vi "Argos 2.0.vi"(0 "PID 1 COM":refnum<visa-resource-name>="COM1", 1 "Setpoint\n START":bool, 2 "Write to File":bool, 3 "SP 1 input (°C)":dbl=10.0 min=0.0 max=1300.0, 4 "Intervall (s)":u32=1 max=600, 5 "Write/\nRead":bool=TRUE, 6 "Delay (ms)":u32=500 min=100 max=600000, 7 "Auto Tune":bool, 9 "Standby":bool, 11 "Reset\nSTOP":bool, 12 "ON":bool=TRUE caption="OFF", 13 "Get Values":bool, 15 "File Path":path) -> (8 "(°C)":dbl format="%#.3f", 14 "SP 1 is (°C)":dbl)   [LabVIEW 2013]
doc: "1. Verwendung\n\nDas Programm dient der Steuerung und Abfrage des Thermocontrollers I3252 und dem Auslesen von zwei VC 840 Messgeräten und einem Druckmessgerät Pfeiffer Single Gauge. \nDie Messgeräte werden Standardmäßig ausgelesen und erst nach Betätigung des Schalters \"Write to File\" in einer Textdatei abgespeichert. Das Eingabefeld \"Intervall\" legt den Abstand der Messpunkte fest.\nDer Setpoint für den Thermocontroller wird erst nach Betätigung des Tasters \"Setpoint START\" übernommen und angesteuert. Er wird ind den EEPROM des Gerätes geschrieben. Die Regelung kann mit Hilfe des Schalters \"Standby\" unterbrochen werden. Durch den Taster \"Reset STOPP\" kann der Setpoint aus dem EEPROM gelöscht werden.\nDie Eingabeflächen \"Constant\" und \"Thickness\" dienen der Berechnung des spezifischen Widerstands.\nDie Eingabeflächen \"User\" und \"Sample\" werden in den Header der Textdatei übernommen.\nDer Indikator \"File Path\" zeigt den aktuellen Speicherort der Textdatei an. Dieser wird nach ausschalten des Schalters \"Write to File\" gelöscht. Bei erneuten Schreiben muss ein neuer Speicherort gewählt werden. Bei Wahl desselben Speicherorts werden sämtliche bereits gespeicherte Daten gelöscht.\n\n\n2. Erläuterungen zum Blockdiagramm\n2.1 äußere Sequenz\nDie äußerte Sequenz besteht aus fünf Frames. Der erste dient der Initialisierung der Ports. Der zweite dient als Verzögerung um dem Programm genug Zeit zu geben die Ports zu öffnen. Jedoch senden die beiden VC 840 bereits Informationen an den Computer die in einem Puffer zwischengespeichert werden. Im dritten Frame wird dieser Puffer geleert. Somit kommt es zu keinem Framing Error. Desweiteren wird in diesem Frame die Startzeit der Messungen genommen. Im vierten Frame wird die eigentliche Messung und Verarbeitung der Daten durchgeführt. Die while-Schleife wird nur durch Auftreten eines Fehlers oder durch Betätigung des Stopbuttons auf dem Front Panel in der oberen linken Ecke unterbrochen. Im fünften und letzten Frame werden die Ports wieder geschlossen und beim Auftreten eines Fehlers wird das Programm automatisch gestoppt. Falls kein Fehler auftritt wird die Sequenz von vorne abgearbeitet.\n\n2.2 while-Schleife und innere Sequenz\n2.2.1 \"Event Structure\"\n2.2.1.1 Allgemein\nDer erste Frame beinhaltet ein \"Event Structure\". Dieser reagiert auf insgesamt elf verschiedene Ereignisse. Falls keines dieser Ereignisse auftreten sollte, warte die Struktur eine Millisekunde bevor die \"Event Structure\" verlassen wird. Die übrigen Ereignisse treten ein, wenn der entsprechende Kontroller eine Werteänderung erfährt.\n\n2.2.1.2 Event: Setpoint\nDieser Case besteht von außen nach innen aus einer Stacked Sequence, einer for-Loop und einer Flat Sequence die wiederum zwei \"Case Structures\" enthält. Als erstes wird bei dem Schalter \"Setpoint START\" der Blinkmodus aktiviert und bei dem Schalter \"Read Temperature\" deaktiviert. Danach folgt das eigentliche setzen des Temperatursollwerts. In der ersten Iteration wird dem Controller I3252 ein Schreibbefehl gesendet. Theoretisch kann der Setpoint in den RAM oder in den EEPROM geschrieben werden. Diese Auswahl erfolgt mit Hilfe des Schalters \"RAM\". Da das Schreiben in den RAM -Speicher aber aus diversen Gründen nicht erwünscht ist, wurde es nicht implementiert. Eine nachträgliche Implementierung ist aber leicht möglich, in dem die untere String-Konstante \"*P012\" durch \"*W012\" ersetzt wird. An diesem Befehl wird eine fünfstellige Hexadezimalzahl angehängt, die den Sollwert wiedergibt. Der Sollwert wird vorher mit zehn multipliziert, da das Komma standardmäßig nach der ersten Ziffer festgesetzt wurde (Bsp.: 800 wird gesendet um 80 einzustellen). Dieser Befehlsstrang wird an das Gerät mittels des SubVIs \"Comm_Interface\", auf welches später noch näher eingegangen wird, weitergegeben. Der durch das Gerät zurückgegebene String wird nicht verarbeitet.\nDie zweite Iteration dient dem Auslesen des eingestellten Sollwertes. Wahlweise kann der RAM- oder der EEPROM-Speicher ausgelesen werden. Die eigentliche Verarbeitung des Ausgabestrings erfolgt durch das SubVI \"Edit Setpoint\".\nDie Implementierung zur Einstellung des zweiten Setpoints erfolgt durch kopieren der ersten beiden Fälle und ersetzen der \"1\" im Befehf durch eine \"2\" (Bsp.: \"*P012\" zu \"*P022\"). Es darf aber nicht vergessen werden, dass dann ebenfalls die Anzahl der Iterationen angepasst werden muss.\nAls letztes wird der Blinkmodus des Schalters \"Setpoint START\" wieder deaktiviert.\n\n2.2.1.3 Event: Standby\nDieses Ereignis aktiviert bzw. deaktiviert als erstes den Blinckmodus des entsprechenden Schalters und sendet danach den Befehl zum aktivieren (\"*D03\") oder zum deaktivieren (\"*E03\") des Standbymodus an den Thermocontroller.\n\n2.2.1.4 Event: Set Command \nDer in das Feld \"Command shall be\" eingegebene Befehl wird an den Thermocontroller übermittlet. Die korrekte Form des Befehls ist im \"Communication Manuel\" nachzuschlagen. Das \"*\"-Zeichen wurde allerdings schon implementiert und muss somit nicht mit eingegeben werden.\n\n2.2.1.5 Event: Reset\nIn der ersten Iteration wird der Reset-Befehl an den Thermocontroller gesendet. In Folge wird der gesamte EEPROM-Speicher gelöscht. Deshalb wird in der zweiten Iteration der Setpoint aktualisiert. Dieser Befehl hat keinen Einfluss auf den RAM-Speicher. Die anschließende Wartezeit ist auf vier Sekunden festgesetzt und wurde empirisch ermittelt. Diese Zeit benötigt das Gerät um den Reset durchzuführen und für die Kommunikation wieder zur Verfügung zu stehen.\n\n2.2.1.6 Event: Auto Tune\nEs ist festgeschrieben, dass der Setpoint für die \"Auto Tune\"-Funktion wenigstens 20°C über der aktuellen Temperatur liegt. Deshalb wird zunächst der aktuelle Temperaturwert ausgelesen. Im zweiten Schritt werden zu diesem Wert zwanzig addiert und der Setpoint wird in den RAM-Speicher geschrieben. Das Schreiben in diesen Speicher ist nötig, da die \"Auto Tune\"-Funktion\" erst nach einem Reset startet. Im dritten Schritt wird der eigentliche Befehl für den \"Auto Tune\" gesendet (siehe dazu \"Communication Manuel\" S.27). Als vierte und letzte Iteration der for-Schleife folgt der bereits erwähnte Reset-Befehl. Der Temperatursollwert, der im RAM-Speicher eingetragen ist, muss zum Schluss wieder auf 0°C gesetzt werden. Die Zeit für die Ausführung des \"Auto Tune\"-Befehls wurde empirisch ermittelt und 45 s festgesetzt.\n\n2.2.1.7 Event: Write LOW/HI\nDieses Ereignis setzt die am Analogausgang anliegende Spannung fest. Normalerweise beträgt dieser Spannungswert 0-10 V. Das angeschlossene Netzteil verträgt aber maximal nur 2,3 V. Aus diesem Grund wird der \"%HIGH\" auf 23 gesetzt. Somit beträgt die maximal anliegende Spannung nur noch 23% von der maximal möglichen, d.h 2,3V. Ein niedrigerer Wert ist jederzeit möglich, genauso wie ein höherer für den Parameter \"%LOW\". Diese werden zunächst nacheinander in den RAM-Speicher geschrieben und anschließend wieder ausgelesen.\n\n2.2.1.8 Event: Set PID\nDie Werte für den PID-Regler können sowohl mit Hilfe der \"Auto Tune\"-Funktion, als auch manuell eingestellt werden. Es wird wiederum zwischen dem Schreiben in den RAM- und dem EEPROM-Speicher unterschieden. Zunächst werden die Werte für \"P\", \"I\" und \"D\", in dieser Reihenfolge, gesetzt und danach die aktuellen Werte ausgelesen.\n\n2.2.1.9 Event: Get Values\nDieses Ereignis hat zur Folge, dass die Werte für \"P\", \"I\", \"D\", \"%LOW\", \"%HIGH\" und des Setpoints wahlweise aus dem RAM- oder EEPROM-Speicher gelesen werden. Die aktuellen Werte werden nicht nur in die entsprechenden Anzeigefelder übernommen, sondern auch in die entsprechenden Eingabefelder, mit Ausnahme des Temperatursollwerts. \n\n2.2.1.10 Event: RAM\nPrinzipiell kann zwischen dem Schreiben in den RAM- oder EEPROM-Speicher des Thermocontrollers gewählt werden. Die entsprechende Schalterposition auf dem Frontpanel zeigt den aktuell verwendeten Speicher an. Die Anzeigewerte werden bei jedem Umschalten aktualisiert und sind im entsprechenden Speicher eingetragen. Die Implementierung ist identisch mit der des Ereignisses \"Get Values\". Es gilt zu beachten, dass die Werte für \"%LOW\" und \"%HIGH\" nur in den RAM-Speicher geschrieben werden können und somit auch nur aus diesem ausgelesen werden können.\n\n2.2.1.11 Event: Set Gauge to Zero\nMit Hilfe der SubVIs \"Get Pressure\" und \"Offset Display\" werden die Werte für den alten und den neuen Offset und der durch den zweiten Drucksensor ermittelt Druck ermittelt. \n\n2.2.1.12 Event: Write to File\nSollte der Schalter \"Write to File\" aktiviert werden, d.h. Schalterposition oben, so wird zunächst durch das SubVI \"Header\" ein Header für die unter \"File Path\" definierte Datei angelegt. Alle Werte, die bereits in der entsprechenden Datei stehen, werden dabei gelöscht.\n\n2.2.2 \"Timed Structures\"\nIm dritten Frame der inneren Sequenz werden die Werte für Zeitpunkt, Temperatur, Spannung, Strom und Druck ermittelt. Damit die Werte zum gleichen Zeitpunkt aufgenommen werden, werden \"Timed Sequences\" eingesetzt. Mit dem entsprechenden Schalter auf dem Front Panel unter dem Tab \"Settings\" kann gewählt werden, ob das entsprechende Gerät ausgelesen werden soll oder nicht. Die einzelnen Sequenzen werden parallel abgearbeitet, womit die Prozesszeit von diesem Frame durch der zeitintensivsten Sequenz abhängt. Dies ist in aller Regel das Auslesen der Temperatur, da ein \"Delay\" von 500 ms oder größer benötigt wird, um den Controller ordentlich ansprechen zu können.\nDie Systemzeit wird durch das SubVI \"System Time in Seconds\" in Sekunden umgerechnet und der in dem Parameter \"Starttime\" gespeicherte Wert wird abgezogen. Somit werden die Sekunden seit dem Start des Programms gezählt.\n\n2.2.3 restlichen Frames\nIm zweiten Frame wird das Intervall zwischen den einzelnen Messwerten festgelegt. Dabei wird der Wert des Parameters \"Delay\" abgezogen. Dieser Wert beträgt im Normalfall 500 ms und ist somit nicht vernachlääsigbar.\nDer Vierte Frame beinhaltet die Umrechnung des Temperatur-Strings in einen Temperaturwert durch das SubVI \"Edit Tmperature\", die Berechnung des spezifischen Widerstands durch das SubVI \"Resistivity Calculation\" und die Überprüfung des Druckwerts. Auch werden die neu gewonnen Werte in das entsprechende Shift-Register übernommen. Falls der Druckwert einen in dem Parameter \"Pressure Limit (mbar)\" festgelegten Grenzwert überschreiten sollte, wird der Thermocontroller automatisch in den Standby-Modus versetzt. Des Weiteren wird der Schalter \"Standby\" solange gesperrt, wie der Druck oberhalb des Grenzwertes liegt. Wenn der Druck wieder unter den Grenzwert gesunken ist, wird der Standby-Befehl nicht automatisch aufgehoben, sondern muss vom Benutzer durch Betätigung des entsprechenden Schalters gegeben werden.\nIm fünften Frame werden die Diagramme erstellt. Dabei wird jedes Mal von neuem das gesamte Shift-Register als Graph dargestellt. Weiterhin werden die Messwerte in ein 1D-Array geschrieben.\nDer sechste und letzte Frame beinhaltet den eigentlich Schreibvorgang der Messwerte in eine Textdatei und die Überprüfung ob ein Fehler vorliegt.\n\n2.3 SubVIs\n2.3.1 Allgemein\nDie SubVIs für die Messgeräte VC840 und das Druckmessgerät wurden aus anderen Quellen übernommen. \n\n2.3.2 \"Header\"\nIn den Header wird zunächst das aktuelle Datum und die aktuelle Zeit übernommen. Die ausgewählte Datei wird dabei überschrieben. Danach wird der Name des Benutzers und der Probe übernommen. Zum Schluss werden die Einheiten in einer Reihe, durch einen Tabulator getrennt, in den Header geschrieben.\n\n2.3.3 \"I3252 Comm Interface\"\nDieses VI stellt die Kommunikation mit dem Thermocontroller her und gibt den Ausgabe-String zurück.\n\n2.3.4 \"I3252 Edit Setpoint\"\nIm Ausgabe-String vom Thermocontroller ist an der vierten Stelle die Stelle des Dezimalpunktes verschlüsselt. Dieses Hexadezimalzahl wird herausgefiltert und an ein \"ENUM Controller\" übergeben. Dieser weist der Hexadezimalzahl eine Nummer zu, mit welcher ein Wert aus einem Array entnommen wird. Dieser Wert dient als Quotient. Der tatsächliche Wert kann somit errechnet werden.\n\n2.3.5 \"I3252 Edit Temperature\"\nDer Temperatur-String, der vom Thermocontroller zurückgegeben wird, wird in eine Dezimalzahl umgewandelt. Manchmal kommt es aus zu Dropouts, die durch dieses Programm herausgefiltert werden. Der letzte Wert wird dabei in einer \"Feedback Node\" gehalten unter der Annahme, dass sich der Temperaturwert nicht sprunghaft ändert.\n\n2.3.6 \"Resistivity Calculation\"\nDer spezifische Widerstand wird nach folgender Formel ausgerechnet. Dabei entspricht t der Dicke der Probe und C ist eine Konstante.\nrho=C*pi*t*U/(ln( 2)*I)\n\n2.3.7 \"System Time in Seconds\"\nZunächst wird die aktuelle Systemzeit ausgelesen. Danach wird diese in Stunden, Minuten und Sekunden aufgeteilt, alles in Sekunden umgerechnet und letztendlich addiert."
uses:
  <vilib>/Platform/TimedLoop/XDataNode/timing_clust.ctl
  <vilib>/Platform/TimedLoop/XDataNode/nitl_modes.ctl
  <vilib>/Platform/TimedLoop/XDataNode/wakeup.ctl
  <vilib>/Instr/_visa.llb/VISA Configure Serial Port (Instr).vi
  <vilib>/Platform/TimedLoop/scheduler/LVUserAPI/_suppVIs/Create_1kHz_TSource.vi
  <vilib>/Utility/file.llb/Write To Spreadsheet File (DBL).vi
  <vilib>/Platform/TimedLoop/XDataNode/XDataNode.xnode
  <vilib>/Platform/TimedLoop/XDataNode/XDNodeRunTimeDep.lvlib
  Dependencies/Pfeiffer TPG261+262 Single+Dual Gauge/Dual Gauge.lvlib
panel:
  out "Thermocouple (Sample holder 1) 2":cluster{dbl[], dbl[]}(graph)
  out "(°C) 2":dbl format="%#.3f"
  out "appended array":dbl[](array[numeric])
  in  "Tab Control":T1(tab)
  out "SP 2 is (°C)":dbl
  in  "SP 2 input (°C)":dbl=10.0 min=0.0 max=1300.0
  in  "Standby\n2":bool
  in  "Setpoint\n START\n2":bool
  out "Pirani (VVP1 Scroll)":cluster{dbl[], dbl[]}(graph)
  in  "Thickness (nm)":dbl min=0.0
  in  "4PP constant":dbl min=0.0 max=5.0
  in  "Sample":string
  in  "User":string
  out "Thermocouple (Sample holder 1)":cluster{dbl[], dbl[]}(graph)
  out "current time (s)":dbl
  out "data logger intervall (s)":dbl
  out "loop time (s)":dbl
  in  "stop":bool
  out "CMR275 Baratron":cluster{dbl[], dbl[]}(graph)
  out "Pressure Baratron 2":dbl format="%#_4e"
  out "PKR251 FullRange":cluster{dbl[], dbl[]}(graph)
  out "Pressure FullRange 2":dbl format="%#_3e"
  out "Pressure Pirani 2":dbl format="%#_3e"
  in  "Reset\nSTOP 2":bool
  out "Pressure OpenPort":cluster{dbl[], dbl[]}(graph)
  out "Pressure OpenPort2":dbl caption="current"
  out "% HIGH Istwert 2":u32
  out "% LOW Istwert 2":u32
  in  "% High Sollwert 2":u32=23 max=24
  in  "% LOW Sollwert 2":u32 max=25
  in  "RAM 2":bool=TRUE caption="EEPROM"
  out "D (Rate) IstWert 2":u32
  out "I ( Reset1) Istwert 2":u32
  out "P (PB1) Istwert 2":u32 caption="actual value"
  in  "D (Rate) Sollwert 2":u32 max=3999
  in  "I ( Reset1) Sollwert 2":u32 max=3999
  in  "P (PB1) Sollwert 2":u32 caption="set value" max=9999
  in  "ON 2":bool=TRUE caption="OFF"
  in  "PID 2 COM":refnum<visa-resource-name>="COM1"
  in  "Delay (ms) 2":u32=500 min=100 max=600000
  in  "Write/\nRead \n\n2":bool=TRUE
  out "status 2":bool caption="Status"
  out "code 2":i32 caption="Code"
  out "code":i32 caption="Code"
  out "status":bool caption="Status"
  in  "Set Gauge to Zero":bool
  out "Status Gauge 1#2":i32(ring) items=["data OK", "underrange", "overrange", "sensor error", "sensor off", "no sensor", "ID error"]
  out "Pressure Gauge 1#2":dbl format="%.3e"
  out "Pressure Gauge 1#1":dbl format="%.3e"
  out "Status Gauge 1#1":i32(ring) items=["data OK", "underrange", "overrange", "sensor error", "sensor off", "no sensor", "ID error"]
  in  "TPG 1 COM":refnum<visa-resource-name>="COM5"
  in  "Pressure Limit (mbar)":dbl=1.0 min=0.0 max=1100.0
  out "Current Offset (mbar)":dbl
  in  "ON (TPG 2)":bool=TRUE caption="OFF"
  in  "ON (TPG 1)":bool=TRUE caption="OFF"
  in  "ON":bool caption="OFF"
  in  "VC 840 2":refnum<visa-resource-name>="COM7"
  out "Reading 2":dbl format="%_4f"
  out "Mode 2":enum16{"?", "Diode", "Beep", "DC", "AC"}(ring)
  out "Unit 2":string
  in  "VC 840 1":refnum<visa-resource-name>="COM7"
  out "Reading 1":dbl format="%_4f"
  out "Mode 1":enum16{"?", "Diode", "Beep", "DC", "AC"}(ring)
  out "Unit 1":string
  out "Status 1":T2
  out "Status 2":T2
  in  "ON":bool caption="OFF"
  out "% HIGH Istwert":u32
  out "% LOW Istwert":u32
  in  "% High Sollwert":u32=23 max=24
  in  "% LOW Sollwert":u32 max=25
  in  "RAM":bool=TRUE caption="EEPROM"
  out "D (Rate) IstWert":u32
  out "I ( Reset1) Istwert":u32
  out "P (PB1) Istwert":u32 caption="actual value"
  in  "D (Rate) Sollwert":u32 max=3999
  in  "I ( Reset1) Sollwert":u32 max=3999
  in  "P (PB1) Sollwert":u32 caption="set value" max=9999
  in  "Set Command":bool
  in  "Set PID":bool
  in  "Write LOW/HI":bool
  out "Command output":string
  in  "Command input":string
  in  "TPG 2 COM":refnum<visa-resource-name>="COM6"
  out "Pressure Gauge 2#2":dbl format="%.3e"
  out "Pressure Gauge 2#1":dbl format="%.3e"
  out "Status Gauge 2#2":i32(ring) items=["data OK", "underrange", "overrange", "sensor error", "sensor off", "no sensor", "ID error"]
  out "Status Gauge 2#1":i32(ring) items=["data OK", "underrange", "overrange", "sensor error", "sensor off", "no sensor", "ID error"]
  out "Command output 2":string
  in  "Command input 2":string
  in  "Set Command\n\n 2":bool
  in  "Auto Tune 2":bool
  in  "Set PID 2":bool
  in  "Write LOW/HI 2":bool
  in  "Get Values 2":bool
  out "Current":cluster{dbl[], dbl[]}(graph)
  out "Voltage":cluster{dbl[], dbl[]}(graph)
  out "Voltage (V)":dbl format="%.4e"
  out "Current (A)":dbl format="%.4e"
  out "Resistivity":cluster{dbl[], dbl[]}(graph)
  out "Resistivity (Ohm*cm)":dbl format="%.3e"
  # "PID 1"
  # "set \nvalue"
  # "actual \nvalue"
  # "T (°C)"
  # "PID 2"
  # "mbar"
  # "Set \nValue\n2"
  # "Actual \nvalue 2"
  # "T (°C)"
  # "mbar"
  # "mbar"
  # "mbar"
  # "Pressure Measurement \n(Pfeiffer TPG261)"
  # "PID Controller (Omega Newport i3252)"
  # "PID Controller 2 (Omega Newport i3252)"
  # "P"
  # "I"
  # "D"
  # "% Low"
  # "% High"
  # "Multimeter\n#1 (VC 840)"
  # "Multimeter\n#2 (VC 840)"
  # "P"
  # "I"
  # "D"
  # "% Low"
  # "% High"
  # "Authors:  Daniel Schuster (sir-dan@web.de)\n                 Steffen Cornelius (s.cornelius@hzdr.de)\n                 Nico Spahn (x)\n\n                 premade SubVIs for readout of Pfeiffer gauge and VC840 Multimeters were used\n                 SubVI \"I3252_Comm_Interface\" is based on a modified Labview example\n\nRelease:  v1.0    \n\nVersion History:\n\nv1.1  -    28.06.2011\n             - Format des Files geändert von %.3f auf %g\n             - maximale Eingabewerte für PID begrenzt\nv1.2  -    12.07.2011\n             - Anzeige p,rho, U, V auf Scientific geändert\n             - y-Achse p,rho auf Log geändert\n             - numerische Zeitanzeige hinzugefügt\n             - 4PP Constant: pi/ln(2)=4,532 set as the default value\nv1.3  -    25.07.2011\n             - Zeitvariable auf EXT geändert, um Sprünge in Diagrammen loszuwerden\nv1.4  -   27.07.2011\n             - ALLE Variablen auf DBL zurückgesetzt wegen Formatierungsproblem im File\n             - Zeitberechnung neu gemacht (Tick count differenzen) -> Zeitsprünge korrigiert ?\n             - Delay/Intervall überarbeitet\nv1.5  -   05.12.2012\n                - Austausch der alten Pfeifer SubvIs durch neue -> nun alle 4 Kanäle des DualGauge\n                                                                                                         Controllers gleichzeitig auslesbar\n                - neue Pfeiffer SubVIs verwendet in Druckwertauslesung und Offset Berechnung des Baratron\n                  Druckes (COM5 Sensor1)\n                - Neuarragement des GUI -> FullRange und Baratron neben Temperatur auf Haupseite zu sehen\n                                                                   Pirani und OpenPort auf Meas.2 zu sehen\n                                                                   Diagnose Seite umfasst nun auch Widerstandsdiagramm\n                - Änderungen der Settingseite -> nun alle 4 Drucksensoren mit aktuellem Messwert und Gerätestatus\n                                                                           zu sehen\n                - The readout of the PID-Temperature Controller and the VC840 Multimeters was not modified\nv1.73  -  18.10.2013\n                - Layout Änderungen\nv.1.8   -  19.01.2014\n                - Änderung Layout Settings Tab\n                - Trennung der beiden TPG Dual Gauge Controls\n                -"
  # "Version 1.73    - last change 18.10.2013"
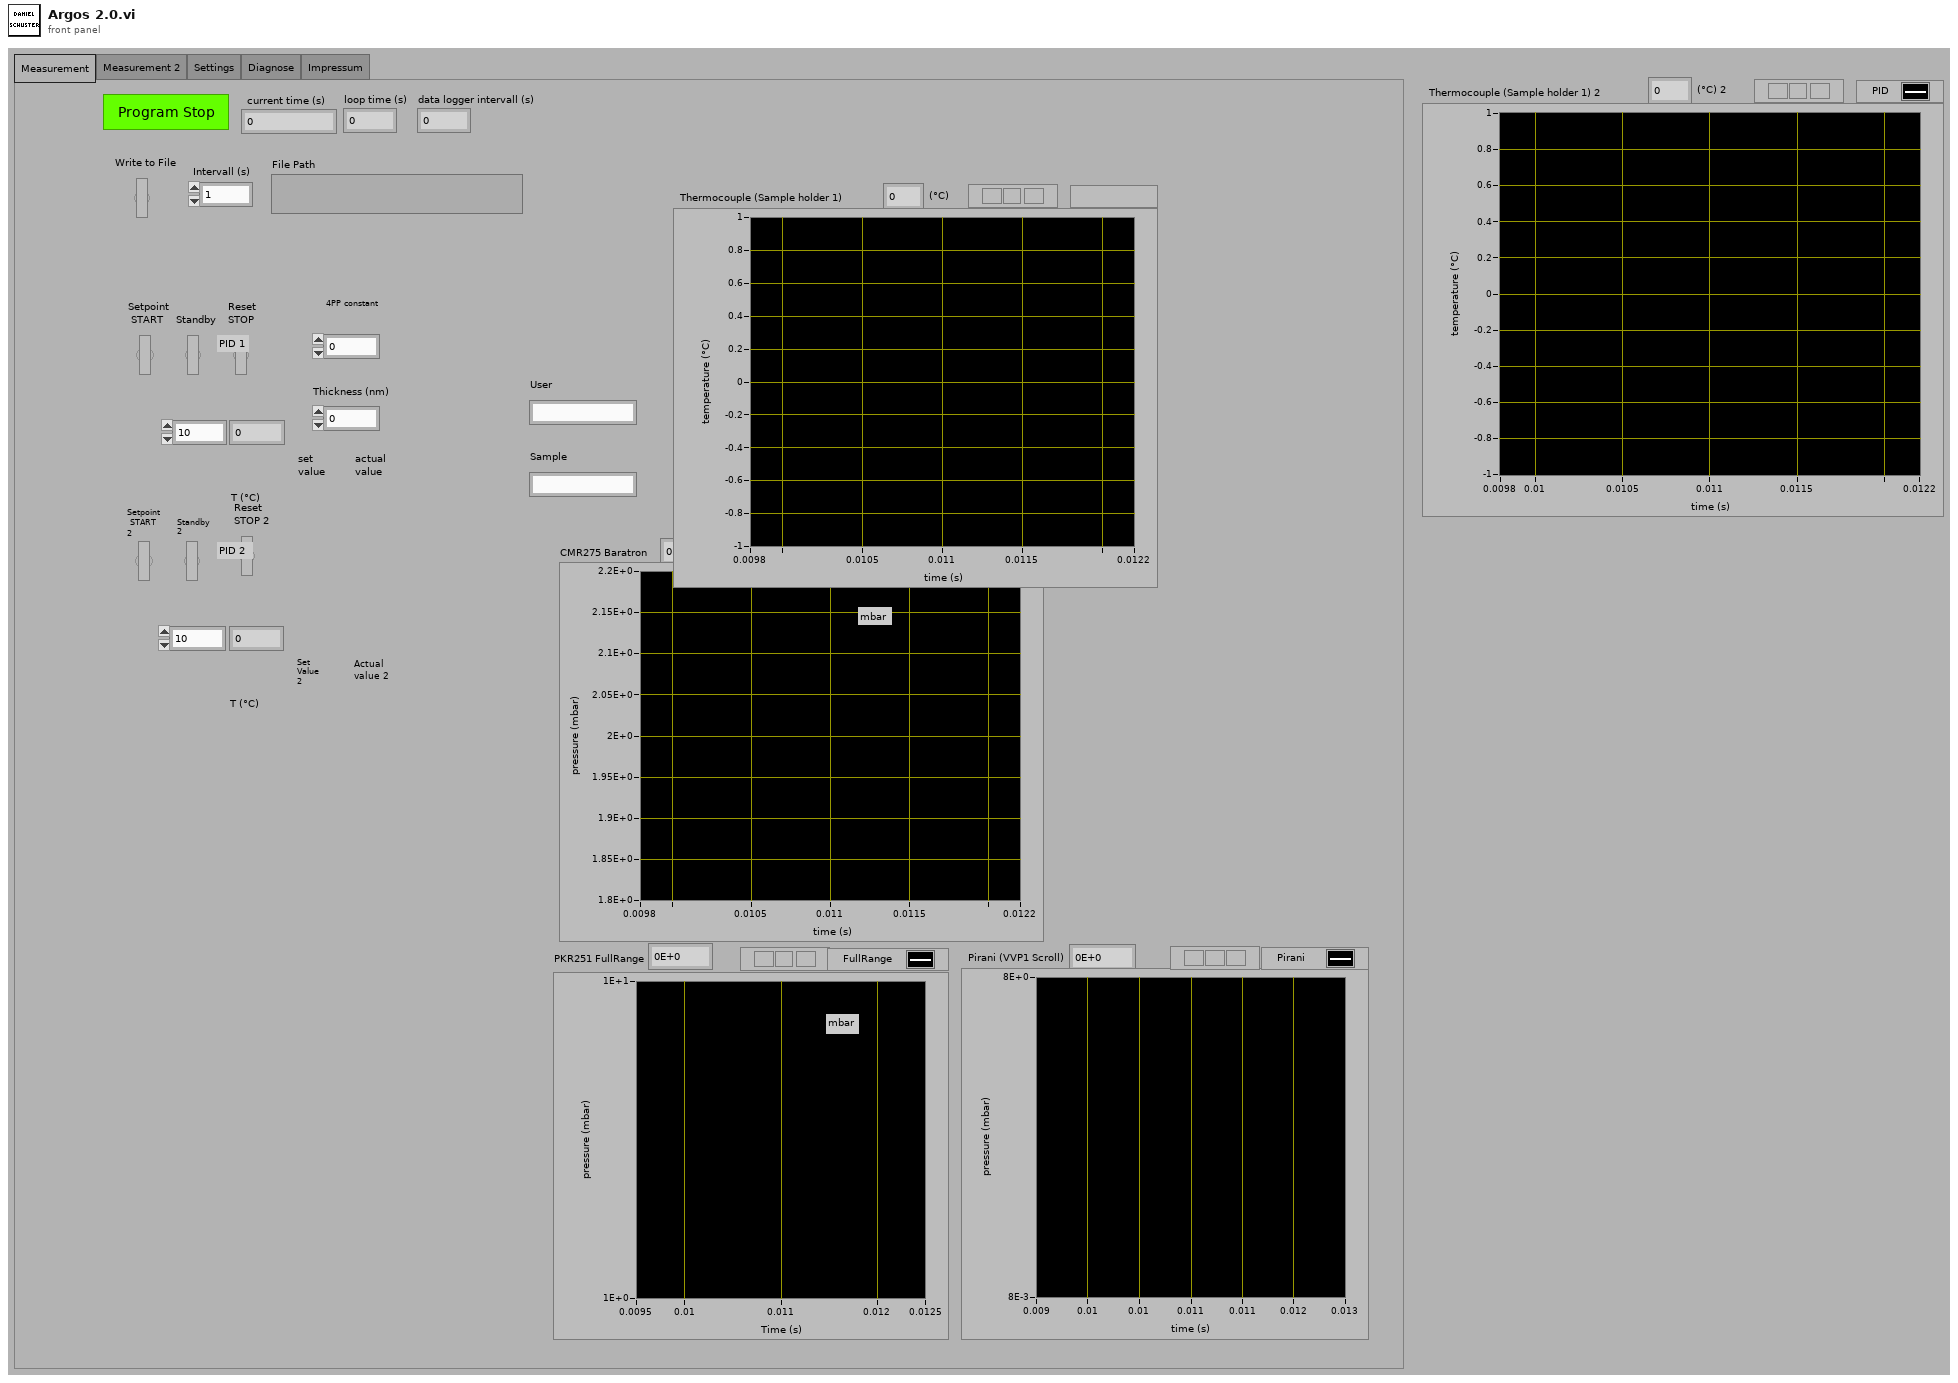
[diagram p1: front panel]
types:
  T1 = enum32{"Measurement", "Measurement 2", "Settings", "Diagnose", "Impressum"}
  T2 = cluster{"Low Bat":bool, "Auto":bool, "Delta":bool, "Hold":bool, "RS232":bool}
  T3 = typedef "XDNodeRunTimeDep.lvlib/timing_clust.ctl" = cluster{"Expected End [f-1]":u64, "Actual End [f-1]":u64, "Finished Late? [f-1]":bool, "Expected End [i-1]":u64, "Actual End [i-1]":u64, "Finished Late? [i-1]":bool, "Expected Start [i]":u64, "Actual Start [i]":u64, "Expected Start [f]":u64, "Actual Start [f]":u64, "Source Name":string, "Structure Name":string, "Period":i64, "Deadline":i64, "Offset":i64, "Start":i64, "Priority":i32, "Timeout":i32, "Mode":T4, "Wakeup Reason":T5, "Error":errorcluster, "Source Type":string, "Secondary Source Type":string, "Global End Time":u64, "Global Start Time":u64, "Frame Duration":u64, "Iteration Duration":u64, "Assigned CPU":i32, "I/O Scan Engine Mode":u32}
  T4 = typedef "XDNodeRunTimeDep.lvlib/nitl_modes.ctl" = enum32{"No Change", "Process missed periods, maintain original phase", "Discard missed periods, maintain original phase", "Process missed periods, ignore original phase", "Discard missed periods, ignore original phase"}
  T5 = typedef "XDNodeRunTimeDep.lvlib/wakeup.ctl" = enum32{"Normal", "Aborted", "Asynchronous wakeup", "Timing source error", "Timed loop error", "Timeout"}
  T6 = enum8{"Enabled", "Disabled", "Disabled and Grayed Out"}
  T7 = cluster{"VISA resource name out":refnum<visa-resource-name>, "error out":errorcluster, "Delay (ms)":u32, "Write/\nRead":bool}
  T8 = cluster{"VISA resource name out":refnum<visa-resource-name>, "error out":errorcluster, "Delay (ms) 2":u32, "Write/\nRead \n\n2":bool}
  T9 = cluster{"TPG 2 COM":refnum<visa-resource-name>, "error out":errorcluster}
  T10 = cluster{"COM out":refnum<visa-resource-name>, "Cluster (Ausgang)":errorcluster}
  T11 = cluster{"Pressure Gauge#1":dbl, "Pressure Gauge#2":dbl}
  T12 = cluster{"TPG 1 COM":refnum<visa-resource-name>, "error out":errorcluster}
  T13 = cluster{"COM out":refnum<visa-resource-name>, "error out":errorcluster, "COM out":refnum<visa-resource-name>, "error out":errorcluster}
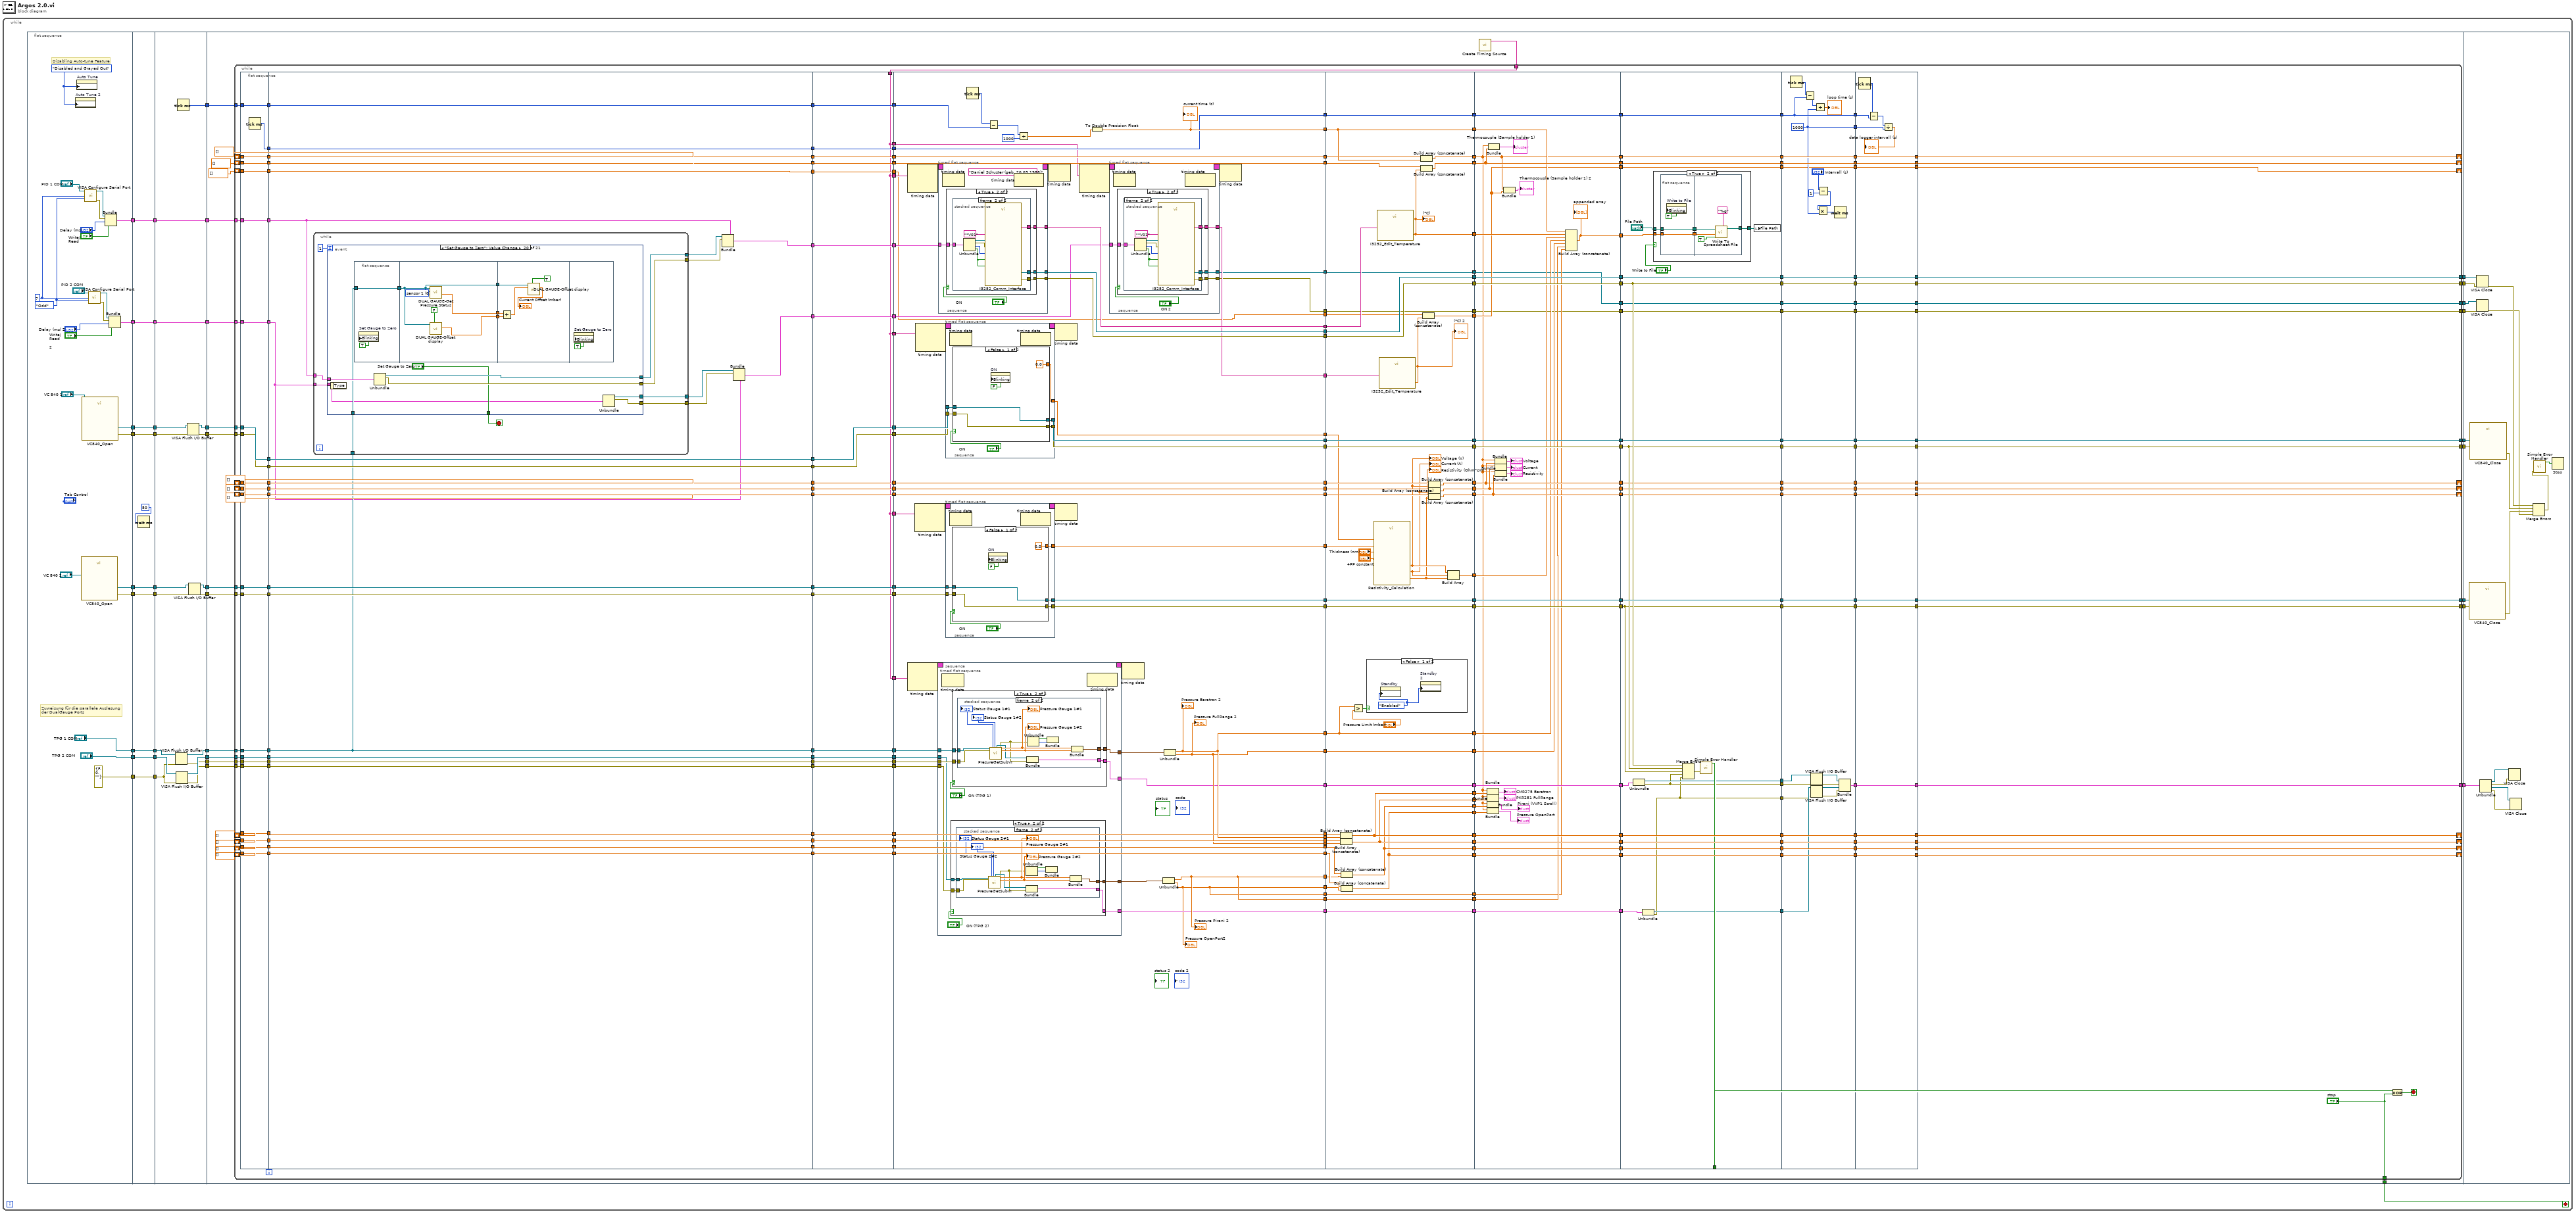
[diagram p0: block diagram]
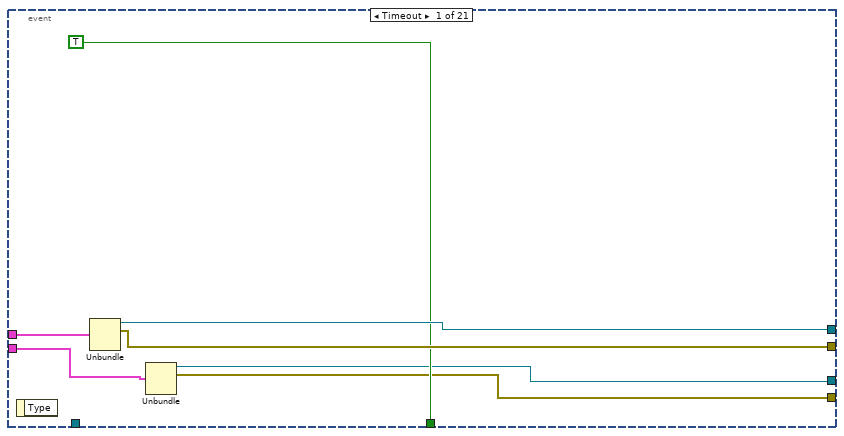
[diagram p2: hidden frame]
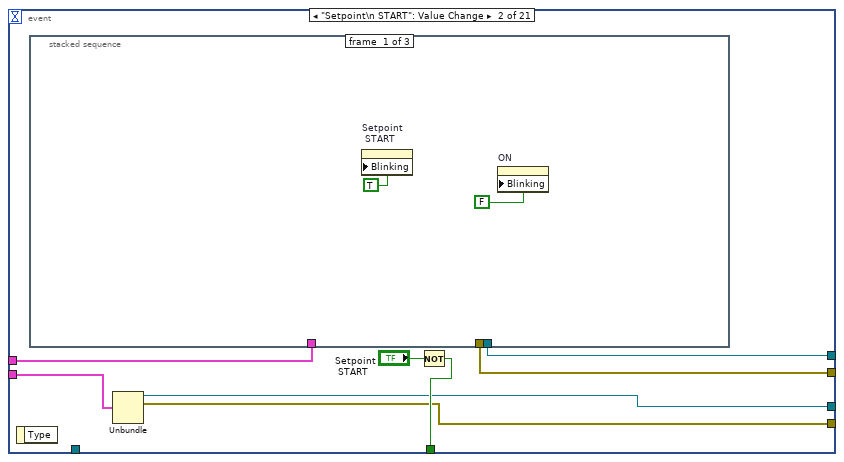
[diagram p3: hidden frame]
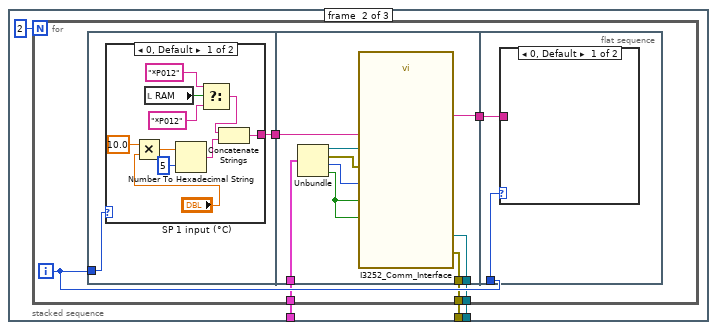
[diagram p4: hidden frame]
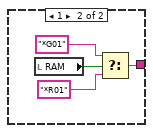
[diagram p5: hidden frame]
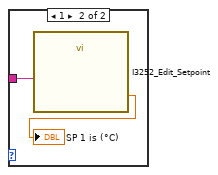
[diagram p6: hidden frame]
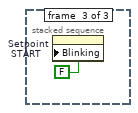
[diagram p7: hidden frame]
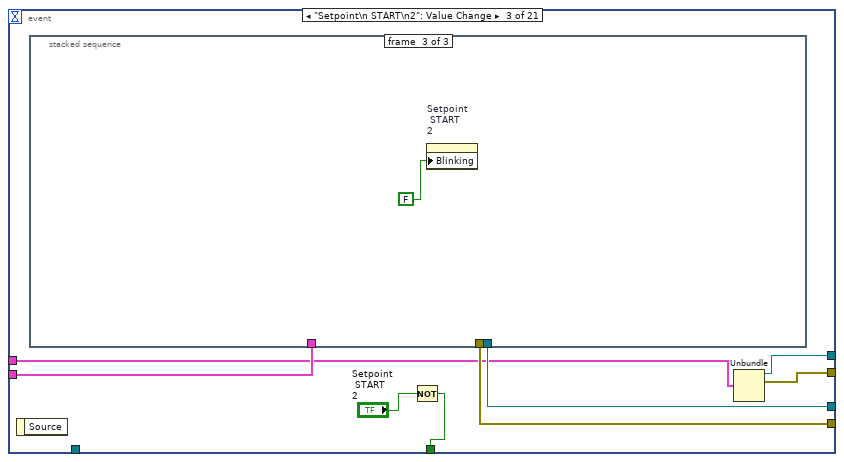
[diagram p8: hidden frame]
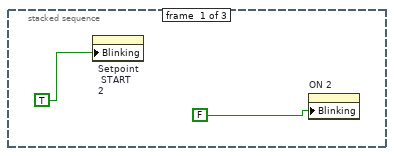
[diagram p9: hidden frame]
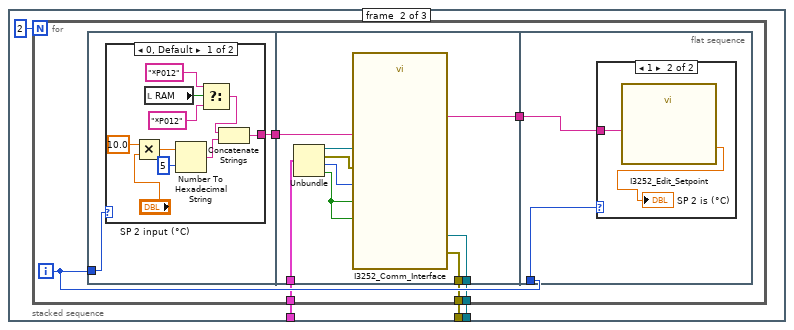
[diagram p10: hidden frame]
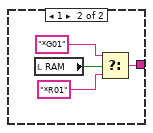
[diagram p11: hidden frame]
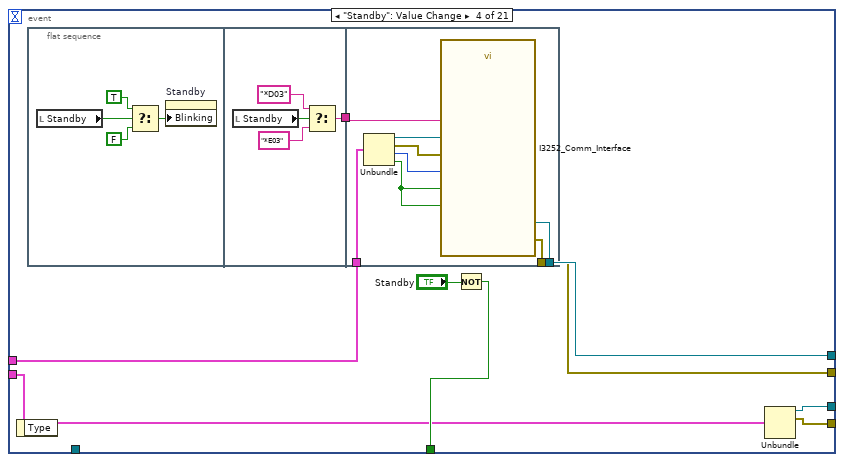
[diagram p13: hidden frame]
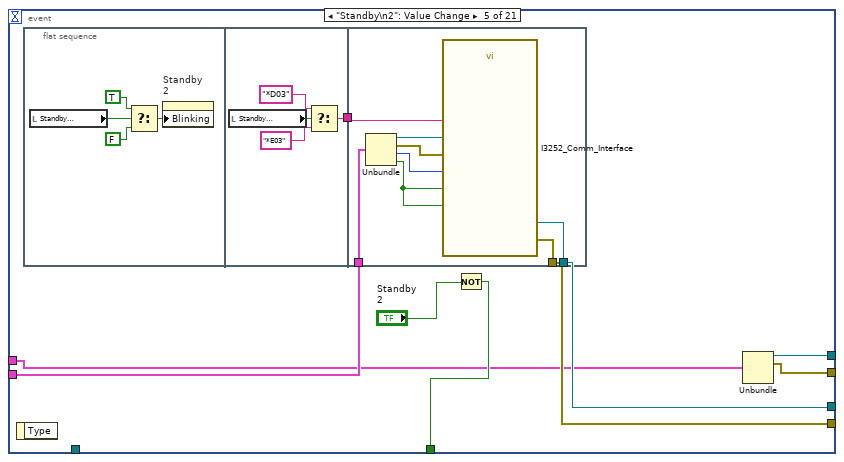
[diagram p14: hidden frame]
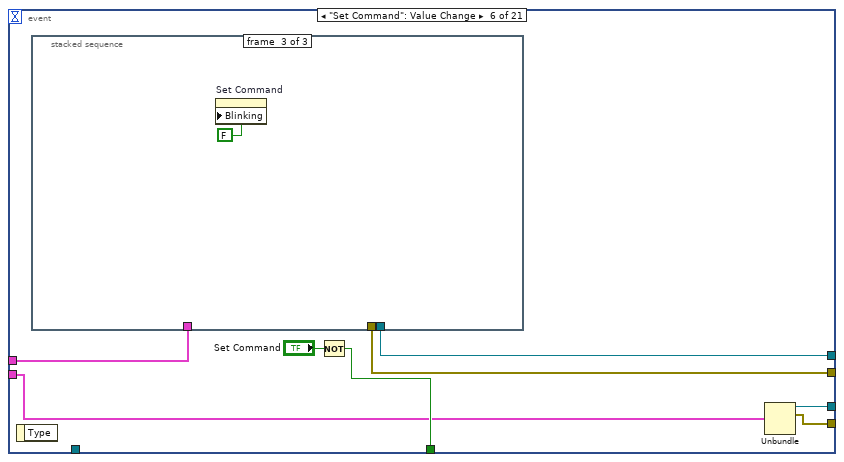
[diagram p15: hidden frame]
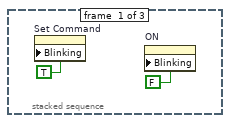
[diagram p16: hidden frame]
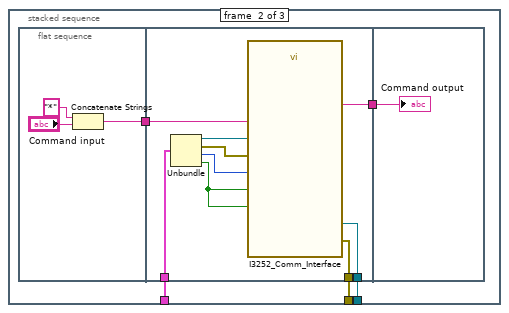
[diagram p17: hidden frame]
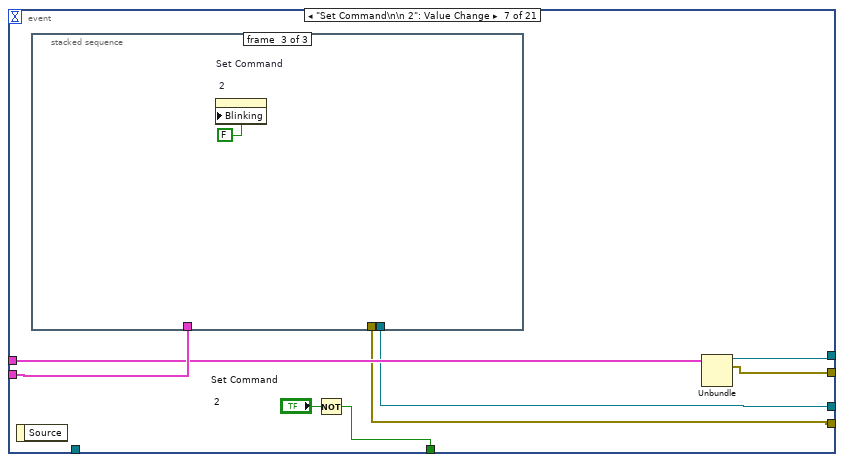
[diagram p18: hidden frame]
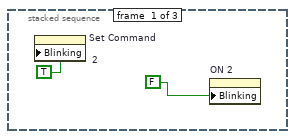
[diagram p19: hidden frame]
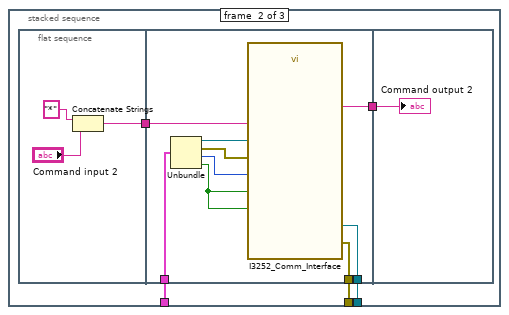
[diagram p20: hidden frame]
diagram:
  n1 = while {
    stop <- w11 stop-if-true
    n2 = flat-sequence {
      tunnel: [w62] -> w39
      tunnel: [w63] -> w38
      tunnel: [w54] -> w37
      tunnel: [w61] -> w36
      tunnel: [w60] -> w35
      tunnel: ["TPG 1 COM"] -> w34
      tunnel: ["TPG 2 COM"] -> w33
      tunnel: [errorcluster {"status"=FALSE, "code"=0, "source"=""} ("Fehler (Eingang)")] -> w8
      tunnel: [w43] -> w3
      tunnel: w39 -> [w73]
      tunnel: [w73] -> w32
      tunnel: w38 -> [w72]
      tunnel: [w72] -> w31
      tunnel: w37 -> [w71]
      tunnel: [w71] -> w30
      tunnel: w36 -> [w70]
      tunnel: [w70] -> w29
      tunnel: w35 -> [w69]
      tunnel: [w69] -> w28
      tunnel: [w67] -> w27
      tunnel: w34 -> [w67]
      tunnel: [w66] -> w26
      tunnel: w33 -> [w66]
      tunnel: [w65] -> w9
      tunnel: w8 -> [w65]
      tunnel: [w64] -> w4
      tunnel: w3 -> [w64]
      tunnel: w32 -> [w85]
      tunnel: [w84] -> w25
      tunnel: w31 -> [w86]
      tunnel: [w83] -> w24
      tunnel: w30 -> [w91]
      tunnel: [w91] -> w23
      tunnel: w29 -> [w88]
      tunnel: [w89] -> w22
      tunnel: w28 -> [w87]
      tunnel: [w90] -> w21
      tunnel: [w82] -> w20
      tunnel: [w80] -> w19
      tunnel: w27 -> [w81]
      tunnel: [w79] -> w18
      tunnel: w26 -> [w78]
      tunnel: w9 -> [w77]
      tunnel: [w76] -> w7
      tunnel: [w75] -> w6
      tunnel: [w74] -> w5
      tunnel: w4 -> [w74]
      tunnel: w25 -> [w123]
      tunnel: w24 -> [w122]
      tunnel: w23 -> [w121]
      tunnel: w22 -> [w119]
      tunnel: w21 -> [w118]
      tunnel: [w117] -> w17
      tunnel: [w116] -> w16
      tunnel: [w115] -> w15
      tunnel: [w114] -> w14
      tunnel: [w113] -> w13
      tunnel: [w112] -> w12
      tunnel: w20 -> [w106]
      tunnel: w19 -> [w105]
      tunnel: w18 -> [w104]
      tunnel: [w99] -> w11
      tunnel: [w98] -> w10
      tunnel: w7 -> [w97]
      tunnel: w6 -> [w96]
      tunnel: w5 -> [w95]
      tunnel: [w94] -> w2
      tunnel: [w93] -> w1
      tunnel: w17 -> [w1952]
      tunnel: w16 -> [w1951]
      tunnel: w15 -> [w1954]
      tunnel: w14 -> [w1953]
      tunnel: w13 -> [w1956]
      tunnel: w12 -> [w1955]
      tunnel: w10 -> [w1949]
      tunnel: w2 -> [w1944]
      tunnel: w1 -> [w1943]
      frame #0 {
        w41 = u16 7 ("data bits (8)")
        w40 = enum16{"None", "Odd", "Even", "Mark", "Space"}."Odd" ("parity (0:none)")
        w42 = T6."Disabled and Grayed Out" ("Disabled")
        # "Disabling Auto-tune Feature"
        # "Zuweisung für die parallele Auslesung\nder DualGauge Ports"
        n3 = property on="Auto Tune 2" class="Bool"("DisabledEnum"=w42) -> ()  [unwired: 2 in, 2 out]
        n4 = property on="Auto Tune" class="Bool"("DisabledEnum"=w42) -> ()  [unwired: 2 in, 2 out]
        n5 = call "VC840_Open.vi"("VISA resource name"="VC 840 2") -> ("error out"=w60:errorcluster, "VISA resource name out"=w61:refnum<visa-resource-name>)  [unwired: 1 in, 8 out]
        n6 = call "VC840_Open.vi"("VISA resource name"="VC 840 1") -> ("error out"=w63:errorcluster, "VISA resource name out"=w62:refnum<visa-resource-name>)  [unwired: 1 in, 8 out]
        n7 = call-poly "VISA Configure Serial Port"("VISA resource name"="PID 1 COM", "data bits (8)"=w41, "parity (0:none)"=w40) -> ("VISA resource name out"=w58:refnum<visa-resource-name>, "error out"=w59:errorcluster)  [unwired: 6 in, 5 out]
        n8 = call-poly "VISA Configure Serial Port"("VISA resource name"="PID 2 COM", "data bits (8)"=w41, "parity (0:none)"=w40) -> ("VISA resource name out"=w47:refnum<visa-resource-name>, "error out"=w48:errorcluster)  [unwired: 6 in, 5 out]
        n9 = Bundle("VISA resource name out"=w58, "error out"=w59, "Delay (ms)"="Delay (ms)", "Write/\nRead"="Write/\nRead") -> (w54:T7)  [unwired: 1 in]
        n10 = Bundle("VISA resource name out"=w47, "error out"=w48, "Delay (ms) 2"="Delay (ms) 2", "Write/\nRead \n\n2"="Write/\nRead \n\n2") -> (w43:T8)  [unwired: 1 in]
      }
      frame #1 {
        n11 = Wait (ms)(milliseconds to wait=u32 50) -> ()  [unwired: 1 out]
      }
      frame #2 {
        n12 = VISA Flush I/O Buffer(VISA resource name=w81, error in (no error)=w77) -> (VISA resource name out=w80:refnum<visa-resource-name>, error out=w76:errorcluster)  [unwired: 1 in]
        n13 = VISA Flush I/O Buffer(VISA resource name=w78, error in (no error)=w77) -> (VISA resource name out=w79:refnum<visa-resource-name>, error out=w75:errorcluster)  [unwired: 1 in]
        n14 = Tick Count (ms)() -> (millisecond timer value=w82:u32)
        n15 = VISA Flush I/O Buffer(VISA resource name=w85, error in (no error)=w86) -> (VISA resource name out=w84:refnum<visa-resource-name>, error out=w83:errorcluster)  [unwired: 1 in]
        n16 = VISA Flush I/O Buffer(VISA resource name=w88, error in (no error)=w87) -> (VISA resource name out=w89:refnum<visa-resource-name>, error out=w90:errorcluster)  [unwired: 1 in]
      }
      frame #3 {
        n17 = call-poly <vilib>:"Create Timing Source.vi"() -> ("name (out)"=w120:string)  [unwired: 10 in, 1 out]
        n18 = while {
          tunnel: w123 -> [w370]
          tunnel: w122 -> [w369]
          tunnel: w121 -> [w368]
          tunnel: w120 -> [w361]
          tunnel: w119 -> [w354]
          tunnel: w118 -> [w353]
          tunnel: [w349] -> w117
          tunnel: [w348] -> w116
          tunnel: [w346] -> w115
          tunnel: [w344] -> w114
          tunnel: [w342] -> w113
          tunnel: [w340] -> w112
          shift-right: [w313] -> _
          shift-left: dbl[] [] -> [w318]
          shift-right: [w291] -> _
          shift-left: dbl[] [] -> [w326]
          shift-right: [w315] -> _
          shift-left: dbl[] [] -> [w322]
          shift-right: [w288] -> _
          shift-left: dbl[] [] -> [w325]
          shift-right: [w285] -> _
          shift-left: dbl[] [] -> [w324]
          tunnel: w106 -> [w279]
          tunnel: w105 -> [w235]
          tunnel: w104 -> [w231]
          shift-right: [w189] -> _
          shift-left: dbl[] [] -> [w219]
          shift-right: [w187] -> _
          shift-left: dbl[] [] -> [w217]
          shift-right: [w185] -> _
          shift-left: dbl[] [] -> [w215]
          shift-right: [w183] -> _
          shift-left: dbl[] [] -> [w213]
          tunnel: ["stop"] -> w99
          tunnel: [w177] -> w98
          tunnel: w97 -> [w172]
          tunnel: w96 -> [w170]
          tunnel: w95 -> [w150]
          shift-right: [w142] -> _
          shift-left: dbl[] [] -> [w140]
          tunnel: [w131] -> w94
          tunnel: [w125] -> w93
          stop <- w176 stop-if-true
          n19 = flat-sequence {
            tunnel: w279 -> [w382]
            tunnel: w318 -> [w383]
            tunnel: w322 -> [w384]
            tunnel: w324 -> [w385]
            tunnel: w325 -> [w386]
            tunnel: w326 -> [w387]
            tunnel: w353 -> [w388]
            tunnel: w354 -> [w389]
            tunnel: w368 -> [w390]
            tunnel: w369 -> [w391]
            tunnel: w370 -> [w392]
            tunnel: [w392] -> w278
            tunnel: [w391] -> w277
            tunnel: [w390] -> w276
            tunnel: [w389] -> w275
            tunnel: [w388] -> w274
            tunnel: [w387] -> w273
            tunnel: [w386] -> w272
            tunnel: [w385] -> w271
            tunnel: [w384] -> w270
            tunnel: [w383] -> w269
            tunnel: [w382] -> w268
            tunnel: [w381] -> w250
            tunnel: [w380] -> w236
            tunnel: w235 -> [w380]
            tunnel: [w379] -> w232
            tunnel: w231 -> [w379]
            tunnel: [w378] -> w220
            tunnel: w219 -> [w378]
            tunnel: [w377] -> w218
            tunnel: w217 -> [w377]
            tunnel: [w376] -> w216
            tunnel: w215 -> [w376]
            tunnel: [w375] -> w214
            tunnel: w213 -> [w375]
            tunnel: [w374] -> w173
            tunnel: w172 -> [w374]
            tunnel: [w373] -> w171
            tunnel: w170 -> [w373]
            tunnel: [w372] -> w151
            tunnel: w150 -> [w372]
            tunnel: [w371] -> w141
            tunnel: w140 -> [w371]
            tunnel: [w420] -> w367
            tunnel: [w419] -> w365
            tunnel: [w415] -> w363
            tunnel: [w414] -> w358
            tunnel: [w413] -> w356
            tunnel: [w412] -> w323
            tunnel: [w411] -> w319
            tunnel: [w410] -> w299
            tunnel: [w409] -> w296
            tunnel: [w408] -> w294
            tunnel: [w407] -> w280
            tunnel: w278 -> [w420]
            tunnel: w277 -> [w419]
            tunnel: w276 -> [w418]
            tunnel: w275 -> [w414]
            tunnel: w274 -> [w413]
            tunnel: w273 -> [w410]
            tunnel: w272 -> [w409]
            tunnel: w271 -> [w408]
            tunnel: w270 -> [w412]
            tunnel: w269 -> [w411]
            tunnel: w268 -> [w407]
            tunnel: [w406] -> w251
            tunnel: w250 -> [w406]
            tunnel: w236 -> [w404]
            tunnel: [w404] -> w233
            tunnel: w232 -> [w405]
            tunnel: [w405] -> w229
            tunnel: w220 -> [w403]
            tunnel: w218 -> [w402]
            tunnel: w216 -> [w401]
            tunnel: w214 -> [w400]
            tunnel: [w403] -> w212
            tunnel: [w402] -> w208
            tunnel: [w401] -> w205
            tunnel: [w400] -> w204
            tunnel: w173 -> [w399]
            tunnel: w171 -> [w398]
            tunnel: [w399] -> w168
            tunnel: [w398] -> w166
            tunnel: w151 -> [w394]
            tunnel: [w393] -> w148
            tunnel: w141 -> [w397]
            tunnel: [w397] -> w139
            tunnel: w367 -> [w1471]
            tunnel: [w1471] -> w366
            tunnel: w365 -> [w1470]
            tunnel: [w1470] -> w364
            tunnel: w363 -> [w1467]
            tunnel: [w1467] -> w362
            tunnel: w361 -> [w1449]
            tunnel: [w1449] -> w360
            tunnel: [w1449] -> w359
            tunnel: w358 -> [w1469]
            tunnel: [w1469] -> w357
            tunnel: w356 -> [w1468]
            tunnel: [w1468] -> w355
            tunnel: [w1449] -> w352
            tunnel: [w1449] -> w338
            tunnel: w323 -> [w1466]
            tunnel: [w1466] -> w321
            tunnel: w319 -> [w1465]
            tunnel: [w1465] -> w316
            tunnel: [w1464] -> w300
            tunnel: w299 -> [w1464]
            tunnel: [w1463] -> w297
            tunnel: w296 -> [w1463]
            tunnel: [w1462] -> w295
            tunnel: w294 -> [w1462]
            tunnel: [w1461] -> w281
            tunnel: w280 -> [w1461]
            tunnel: [w1460] -> w252
            tunnel: w251 -> [w1460]
            tunnel: [w1459] -> w234
            tunnel: w233 -> [w1459]
            tunnel: [w1458] -> w230
            tunnel: w229 -> [w1458]
            tunnel: w212 -> [w1457]
            tunnel: [w1457] -> w211
            tunnel: [w1456] -> w209
            tunnel: w208 -> [w1456]
            tunnel: [w1455] -> w207
            tunnel: w205 -> [w1455]
            tunnel: w204 -> [w1454]
            tunnel: [w1454] -> w203
            tunnel: [w1453] -> w169
            tunnel: w168 -> [w1453]
            tunnel: [w1452] -> w167
            tunnel: w166 -> [w1452]
            tunnel: [w1451] -> w149
            tunnel: w148 -> [w1451]
            tunnel: w139 -> [w1450]
            tunnel: [w1450] -> w138
            tunnel: [w1449] -> w124
            tunnel: [w1502] -> w337
            tunnel: w366 -> [w1531]
            tunnel: w364 -> [w1530]
            tunnel: w362 -> [w1527]
            tunnel: w360 -> [w1526]
            tunnel: w359 -> [w1525]
            tunnel: w357 -> [w1515]
            tunnel: w355 -> [w1514]
            tunnel: w352 -> [w1516]
            tunnel: [w1512] -> w336
            tunnel: [w1513] -> w335
            tunnel: [w1524] -> w334
            tunnel: [w1523] -> w333
            tunnel: [w1522] -> w332
            tunnel: [w1521] -> w331
            tunnel: w338 -> [w1511]
            tunnel: [w1510] -> w330
            tunnel: [w1509] -> w329
            tunnel: [w1493] -> w328
            tunnel: [w1508] -> w327
            tunnel: w321 -> [w1507]
            tunnel: [w1507] -> w320
            tunnel: [w1506] -> w317
            tunnel: w316 -> [w1506]
            tunnel: w300 -> [w1505]
            tunnel: [w1505] -> w298
            tunnel: w297 -> [w1504]
            tunnel: w295 -> [w1503]
            tunnel: [w1504] -> w293
            tunnel: [w1503] -> w292
            tunnel: w281 -> [w1501]
            tunnel: [w1497] -> w253
            tunnel: w252 -> [w1497]
            tunnel: w234 -> [w1495]
            tunnel: w230 -> [w1494]
            tunnel: [w1488] -> w228
            tunnel: [w1493] -> w227
            tunnel: [w1491] -> w226
            tunnel: [w1489] -> w225
            tunnel: w211 -> [w1492]
            tunnel: [w1492] -> w210
            tunnel: w209 -> [w1491]
            tunnel: w207 -> [w1490]
            tunnel: [w1490] -> w206
            tunnel: w203 -> [w1489]
            tunnel: [w1488] -> w181
            tunnel: [w1487] -> w178
            tunnel: w169 -> [w1486]
            tunnel: w167 -> [w1485]
            tunnel: [w1482] -> w162
            tunnel: [w1480] -> w161
            tunnel: [w1482] -> w160
            tunnel: [w1481] -> w156
            tunnel: [w1480] -> w153
            tunnel: w149 -> [w1477]
            tunnel: [w1476] -> w147
            tunnel: w138 -> [w1475]
            tunnel: [w1475] -> w137
            tunnel: [w1474] -> w135
            tunnel: [w1473] -> w126
            tunnel: w124 -> [w1472]
            tunnel: w337 -> [w1778]
            tunnel: [w1775] -> w311
            tunnel: w336 -> [w1791]
            tunnel: [w1791] -> w310
            tunnel: w335 -> [w1790]
            tunnel: [w1790] -> w309
            tunnel: w334 -> [w1789]
            tunnel: [w1789] -> w308
            tunnel: w333 -> [w1788]
            tunnel: [w1788] -> w307
            tunnel: w332 -> [w1787]
            tunnel: [w1787] -> w306
            tunnel: w331 -> [w1786]
            tunnel: [w1786] -> w305
            tunnel: [w1779] -> w304
            tunnel: w330 -> [w1772]
            tunnel: w329 -> [w1780]
            tunnel: w328 -> [w1779]
            tunnel: w327 -> [w1781]
            tunnel: [w1778] -> w303
            tunnel: w320 -> [w1777]
            tunnel: w317 -> [w1776]
            tunnel: [w1774] -> w302
            tunnel: [w1762] -> w301
            tunnel: w298 -> [w1773]
            tunnel: w293 -> [w1770]
            tunnel: w292 -> [w1769]
            tunnel: [w1771] -> w289
            tunnel: [w1768] -> w286
            tunnel: [w1767] -> w283
            tunnel: [w1763] -> w282
            tunnel: [w1761] -> w254
            tunnel: w253 -> [w1761]
            tunnel: w228 -> [w1760]
            tunnel: w227 -> [w1759]
            tunnel: w226 -> [w1758]
            tunnel: w225 -> [w1756]
            tunnel: [w1754] -> w224
            tunnel: [w1753] -> w223
            tunnel: [w1752] -> w222
            tunnel: [w1751] -> w221
            tunnel: w210 -> [w1755]
            tunnel: w206 -> [w1757]
            tunnel: [w1754] -> w202
            tunnel: [w1753] -> w201
            tunnel: [w1752] -> w200
            tunnel: [w1751] -> w199
            tunnel: [w1750] -> w182
            tunnel: w181 -> [w1750]
            tunnel: [w1749] -> w179
            tunnel: w178 -> [w1749]
            tunnel: w162 -> [w1748]
            tunnel: w161 -> [w1747]
            tunnel: w160 -> [w1746]
            tunnel: [w1746] -> w159
            tunnel: [w1745] -> w157
            tunnel: w156 -> [w1745]
            tunnel: w153 -> [w1744]
            tunnel: [w1744] -> w152
            tunnel: w147 -> [w1743]
            tunnel: [w1741] -> w146
            tunnel: w137 -> [w1740]
            tunnel: [w1739] -> w136
            tunnel: w135 -> [w1739]
            tunnel: [w1738] -> w127
            tunnel: w126 -> [w1738]
            tunnel: w311 -> [w1829]
            tunnel: [w1836] -> w351
            tunnel: [w1835] -> w350
            tunnel: w310 -> [w1835]
            tunnel: [w1830] -> w347
            tunnel: w309 -> [w1830]
            tunnel: [w1834] -> w345
            tunnel: w308 -> [w1834]
            tunnel: [w1833] -> w343
            tunnel: w307 -> [w1833]
            tunnel: [w1832] -> w341
            tunnel: w306 -> [w1832]
            tunnel: [w1831] -> w339
            tunnel: w305 -> [w1831]
            tunnel: w304 -> [w1818]
            tunnel: w303 -> [w1819]
            tunnel: w302 -> [w1797]
            tunnel: [w1797] -> w314
            tunnel: w301 -> [w1820]
            tunnel: [w1820] -> w312
            tunnel: [w1822] -> w290
            tunnel: w289 -> [w1822]
            tunnel: [w1823] -> w287
            tunnel: w286 -> [w1823]
            tunnel: [w1824] -> w284
            tunnel: w283 -> [w1824]
            tunnel: w282 -> [w1828]
            tunnel: [w1817] -> w255
            tunnel: w254 -> [w1817]
            tunnel: w224 -> [w1814]
            tunnel: w223 -> [w1813]
            tunnel: w222 -> [w1812]
            tunnel: w221 -> [w1811]
            tunnel: w202 -> [w1810]
            tunnel: w201 -> [w1809]
            tunnel: w200 -> [w1808]
            tunnel: w199 -> [w1807]
            tunnel: [w1810] -> w197
            tunnel: [w1809] -> w195
            tunnel: [w1808] -> w193
            tunnel: [w1807] -> w191
            tunnel: w182 -> [w1806]
            tunnel: [w1805] -> w180
            tunnel: w179 -> [w1805]
            tunnel: w159 -> [w1802]
            tunnel: [w1801] -> w158
            tunnel: w157 -> [w1801]
            tunnel: w152 -> [w1800]
            tunnel: w146 -> [w1798]
            tunnel: [w1798] -> w143
            tunnel: w136 -> [w1796]
            tunnel: [w1796] -> w132
            tunnel: [w1795] -> w128
            tunnel: w127 -> [w1795]
            tunnel: w351 -> [w1852]
            tunnel: w350 -> [w1867]
            tunnel: w347 -> [w1861]
            tunnel: w345 -> [w1866]
            tunnel: w343 -> [w1863]
            tunnel: w341 -> [w1865]
            tunnel: w339 -> [w1864]
            tunnel: w314 -> [w1857]
            tunnel: w312 -> [w1856]
            tunnel: w290 -> [w1855]
            tunnel: w287 -> [w1854]
            tunnel: w284 -> [w1853]
            tunnel: [w1846] -> w175
            tunnel: [w1867] -> w267
            tunnel: [w1861] -> w266
            tunnel: [w1866] -> w265
            tunnel: [w1863] -> w264
            tunnel: [w1865] -> w263
            tunnel: [w1864] -> w262
            tunnel: [w1857] -> w261
            tunnel: [w1856] -> w260
            tunnel: [w1855] -> w259
            tunnel: [w1854] -> w258
            tunnel: [w1853] -> w257
            tunnel: [w1851] -> w256
            tunnel: w255 -> [w1851]
            tunnel: [w1850] -> w198
            tunnel: w197 -> [w1850]
            tunnel: [w1849] -> w196
            tunnel: w195 -> [w1849]
            tunnel: [w1848] -> w194
            tunnel: w193 -> [w1848]
            tunnel: [w1847] -> w192
            tunnel: w191 -> [w1847]
            tunnel: w180 -> [w1845]
            tunnel: [w1844] -> w165
            tunnel: [w1843] -> w164
            tunnel: w158 -> [w1842]
            tunnel: [w1841] -> w155
            tunnel: [w1840] -> w154
            tunnel: [w1839] -> w144
            tunnel: w143 -> [w1839]
            tunnel: [w1838] -> w133
            tunnel: w132 -> [w1838]
            tunnel: [w1837] -> w129
            tunnel: w128 -> [w1837]
            tunnel: w267 -> [w1917]
            tunnel: w266 -> [w1916]
            tunnel: w265 -> [w1915]
            tunnel: w264 -> [w1914]
            tunnel: w263 -> [w1913]
            tunnel: w262 -> [w1912]
            tunnel: w261 -> [w1911]
            tunnel: w260 -> [w1910]
            tunnel: w259 -> [w1909]
            tunnel: w258 -> [w1908]
            tunnel: w257 -> [w1907]
            tunnel: w256 -> [w1900]
            tunnel: [w1917] -> w249
            tunnel: [w1916] -> w248
            tunnel: [w1915] -> w247
            tunnel: [w1914] -> w246
            tunnel: [w1913] -> w245
            tunnel: [w1912] -> w244
            tunnel: [w1911] -> w243
            tunnel: [w1910] -> w242
            tunnel: [w1909] -> w241
            tunnel: [w1908] -> w240
            tunnel: [w1907] -> w239
            tunnel: [w1900] -> w238
            tunnel: [w1899] -> w237
            tunnel: w198 -> [w1897]
            tunnel: w196 -> [w1896]
            tunnel: w194 -> [w1895]
            tunnel: w192 -> [w1894]
            tunnel: [w1897] -> w190
            tunnel: [w1896] -> w188
            tunnel: [w1895] -> w186
            tunnel: [w1894] -> w184
            tunnel: w165 -> [w1893]
            tunnel: w164 -> [w1892]
            tunnel: [w1887] -> w163
            tunnel: w155 -> [w1886]
            tunnel: w154 -> [w1885]
            tunnel: [w1884] -> w145
            tunnel: w144 -> [w1884]
            tunnel: [w1883] -> w134
            tunnel: w133 -> [w1883]
            tunnel: [w1882] -> w130
            tunnel: w129 -> [w1882]
            tunnel: [w1931] -> w285
            tunnel: [w1932] -> w288
            tunnel: [w1933] -> w291
            tunnel: [w1934] -> w313
            tunnel: [w1935] -> w315
            tunnel: [w1936] -> w340
            tunnel: [w1937] -> w342
            tunnel: [w1938] -> w344
            tunnel: [w1939] -> w346
            tunnel: [w1940] -> w348
            tunnel: [w1941] -> w349
            tunnel: w249 -> [w1941]
            tunnel: w248 -> [w1940]
            tunnel: w247 -> [w1939]
            tunnel: w246 -> [w1938]
            tunnel: w245 -> [w1937]
            tunnel: w244 -> [w1936]
            tunnel: w243 -> [w1935]
            tunnel: w242 -> [w1934]
            tunnel: w241 -> [w1933]
            tunnel: w240 -> [w1932]
            tunnel: w239 -> [w1931]
            tunnel: w238 -> [w1927]
            tunnel: w237 -> [w1926]
            tunnel: [w1925] -> w189
            tunnel: w190 -> [w1925]
            tunnel: [w1924] -> w187
            tunnel: w188 -> [w1924]
            tunnel: [w1923] -> w185
            tunnel: w186 -> [w1923]
            tunnel: [w1922] -> w183
            tunnel: w184 -> [w1922]
            tunnel: [w1921] -> w177
            tunnel: w163 -> [w1921]
            tunnel: [w1920] -> w142
            tunnel: w145 -> [w1920]
            tunnel: w134 -> [w1919]
            tunnel: [w1919] -> w131
            tunnel: w130 -> [w1918]
            tunnel: [w1918] -> w125
            frame #0 {
              n20 = Tick Count (ms)() -> (millisecond timer value=w381:u32)
            }
            frame #1 {
              n21 = while {
                tunnel: w418 -> [w428]
                tunnel: [w427] -> w417
                tunnel: [w423] -> w416
                tunnel: w404 -> [w425]
                tunnel: w394 -> [w424]
                tunnel: [w422] -> w396
                tunnel: [w421] -> w395
                stop <- w429 stop-if-true
                n22 = event shown="[19] \"Set Gauge to Zero\": Value Change" {
                  selector: _ -> [_ _ _ _ _ _ _ _ _ _ _ _ _ _ _ _ _ _ _ _ _]
                  dyn-events: _ -> [_ _ _ _ _ _ _ _ _ _ _ _ _ _ _ _ _ _ _ _ _]
                  timeout: 1 -> [_ _ _ _ _ _ _ _ _ _ _ _ _ _ _ _ _ _ _ _ _]
                  tunnel: [TRUE ("Set Gauge to Zero") w443 w494 w545 w570 w594 w623 w652 w691 w729 w787 w846 w900 w954 w1036 w1118 w1192 w1266 w1340 "Set Gauge to Zero" _] -> w429
                  tunnel: w428 -> [w436 w442 w489 w542 w564 w592 w620 w648 w686 w728 w782 w842 w898 w952 w1034 w1116 w1188 w1264 w1338 w1418 w1443]
                  tunnel: [w435 w441 w488 w541 w563 w591 w617 w650 w685 w726 w784 w844 w897 w951 w1033 w1115 w1190 w1263 w1337 w1417 w1442] -> w427
                  tunnel: [w434 w440 w487 w540 w562 w590 w616 w649 w684 w727 w783 w843 w896 w950 w1032 w1114 w1189 w1262 w1336 w1416 w1441] -> w423
                  tunnel: w425 -> [_ _ _ _ _ _ _ _ _ _ _ _ _ _ _ _ _ _ _ w1414 _]
                  tunnel: w424 -> [w432 w439 w492 w539 w567 w589 w621 w645 w689 w725 w781 w841 w895 w949 w1029 w1113 w1187 w1261 w1335 w1409 w1435]
                  tunnel: [w430 w438 w491 w538 w566 w588 w619 w647 w688 w724 w786 w840 w894 w948 w1031 w1112 w1186 w1260 w1334 w1408 w1434] -> w422
                  tunnel: [w431 w437 w490 w537 w565 w587 w618 w646 w687 w723 w785 w839 w893 w947 w1030 w1111 w1185 w1259 w1333 w1407 w1433] -> w421
                  event Timeout {
                    n23 = event-data() -> ()  [unwired: 1 in, 1 out]
                    n24 = Unbundle(w436) -> ("VISA resource name out"=w435:refnum<visa-resource-name>, "error out"=w434:errorcluster)  [unwired: 2 out]
                    n25 = Unbundle(w432) -> ("VISA resource name out"=w430:refnum<visa-resource-name>, "error out"=w431:errorcluster)  [unwired: 2 out]
                  }
                  event "Setpoint\n START": Value Change {
                    n26 = event-data() -> ()  [unwired: 1 in, 1 out]
                    n27 = stacked-sequence {
                      tunnel: w442 -> [_ w449 _]
                      tunnel: [_ w448 _] -> w440
                      tunnel: [_ w447 _] -> w441
                      frame #0 {
                        n28 = property on="Setpoint\n START" class="Bool"("Blinking"=TRUE) -> ()  [unwired: 2 in, 2 out]
                        n29 = property on="ON" class="Bool (strict)"("Blinking"=FALSE) -> ()  [unwired: 2 in, 2 out]
                      }
                      frame #1 {
                        n30 = for {
                          N: 2 -> [_]
                          tunnel: w449 -> [w453]
                          tunnel: [w452] -> w448
                          tunnel: [w451] -> w447
                          i -> [w455]
                          n31 = flat-sequence {
                            tunnel: [w458] -> w454
                            tunnel: w455 -> [w457]
                            tunnel: [w476] -> w456
                            tunnel: w454 -> [w475]
                            tunnel: w453 -> [w477]
                            tunnel: [w474] -> w452
                            tunnel: [w473] -> w451
                            tunnel: w456 -> [w483]
                            tunnel: w455 -> [w482]
                            frame #0 {
                              n32 = case shown="0, Default" w457 {
                                tunnel: [w467 w469] -> w458
                                frame 0, Default {
                                n33 = Multiply(x=10.0, y="SP 1 input (°C)") -> (x*y=w464:dbl)
                                n34 = local read "RAM"() -> (w462:bool)
                                n35 = Number To Hexadecimal String(1:i16 5 ("width (-)"), 2:w464) -> (0:w466:string)
                                n36 = Select(t="*P012", s=w462, f="*P012") -> (s? t:f=w459:string)
                                n37 = Concatenate Strings(w459, w466) -> (w467:string)
                                }
                                frame 1 {
                                n38 = local read "RAM"() -> (w472:bool)
                                n39 = Select(t="*G01", s=w472, f="*R01") -> (s? t:f=w469:string)
                                }
                              }
                            }
                            frame #1 {
                              n40 = Unbundle(w477) -> ("VISA resource name out"=w478:refnum<visa-resource-name>, "error out"=w480:errorcluster, "Delay (ms)"=w479:u32, "Write/\nRead"=w481:bool)
                              n41 = call "I3252_Comm_Interface.vi"("VISA resource name in"=w478, "error in"=w480, "Delay (ms)"=w479, "Write"=w481, "String to Write"=w475, "Read"=w481) -> ("VISA resource name out"=w473:refnum<visa-resource-name>, "error out"=w474:errorcluster, "Read String"=w476:string)  [unwired: 2 in]
                            }
                            frame #2 {
                              n42 = case shown="0, Default" w482 {
                                tunnel: w483 -> [_ w485]
                                frame 0, Default {
                                }
                                frame 1 {
                                n43 = call "I3252_Edit_Setpoint.vi"("Read String"=w485) -> ("Setpoint is"=→"SP 1 is (°C)":dbl)
                                }
                              }
                            }
                          }
                        }
                      }
                      frame #2 {
                        n44 = property on="Setpoint\n START" class="Bool"("Blinking"=FALSE) -> ()  [unwired: 2 in, 2 out]
                      }
                    }
                    n45 = Unbundle(w439) -> ("VISA resource name out"=w438:refnum<visa-resource-name>, "error out"=w437:errorcluster)  [unwired: 2 out]
                    n46 = Not(x="Setpoint\n START") -> (.not. x?=w443:bool)
                  }
                  event "Setpoint\n START\n2": Value Change {
                    n47 = event-data() -> ()  [unwired: 1 in, 1 out]
                    n48 = stacked-sequence {
                      tunnel: w492 -> [_ w499 _]
                      tunnel: [_ w498 _] -> w490
                      tunnel: [_ w497 _] -> w491
                      frame #0 {
                        n49 = property on="Setpoint\n START\n2" class="Bool"("Blinking"=TRUE) -> ()  [unwired: 2 in, 2 out]
                        n50 = property on="ON 2" class="Bool (strict)"("Blinking"=FALSE) -> ()  [unwired: 2 in, 2 out]
                      }
                      frame #1 {
                        n51 = for {
                          N: 2 -> [_]
                          tunnel: w499 -> [w503]
                          tunnel: [w502] -> w498
                          tunnel: [w501] -> w497
                          i -> [w505]
                          n52 = flat-sequence {
                            tunnel: [w508] -> w504
                            tunnel: w505 -> [w507]
                            tunnel: [w526] -> w506
                            tunnel: w504 -> [w525]
                            tunnel: w503 -> [w527]
                            tunnel: [w524] -> w502
                            tunnel: [w523] -> w501
                            tunnel: w506 -> [w533]
                            tunnel: w505 -> [w532]
                            frame #0 {
                              n53 = case shown="0, Default" w507 {
                                tunnel: [w517 w519] -> w508
                                frame 0, Default {
                                n54 = Multiply(x=10.0, y="SP 2 input (°C)") -> (x*y=w515:dbl)
                                n55 = local read "RAM"() -> (w513:bool)
                                n56 = Number To Hexadecimal String(1:i16 5 ("width (-)"), 2:w515) -> (0:w516:string)
                                n57 = Select(t="*P012", s=w513, f="*P012") -> (s? t:f=w510:string)
                                n58 = Concatenate Strings(w510, w516) -> (w517:string)
                                }
                                frame 1 {
                                n59 = local read "RAM"() -> (w522:bool)
                                n60 = Select(t="*G01", s=w522, f="*R01") -> (s? t:f=w519:string)
                                }
                              }
                            }
                            frame #1 {
                              n61 = Unbundle(w527) -> ("VISA resource name out"=w528:refnum<visa-resource-name>, "error out"=w530:errorcluster, "Delay (ms) 2"=w529:u32, "Write/\nRead \n\n2"=w531:bool)
                              n62 = call "I3252_Comm_Interface.vi"("VISA resource name in"=w528, "error in"=w530, "Delay (ms)"=w529, "Write"=w531, "String to Write"=w525, "Read"=w531) -> ("VISA resource name out"=w523:refnum<visa-resource-name>, "error out"=w524:errorcluster, "Read String"=w526:string)  [unwired: 2 in]
                            }
                            frame #2 {
                              n63 = case shown="1" w532 {
                                tunnel: w533 -> [_ w535]
                                frame 0, Default {
                                }
                                frame 1 {
                                n64 = call "I3252_Edit_Setpoint.vi"("Read String"=w535) -> ("Setpoint is"=→"SP 2 is (°C)":dbl)
                                }
                              }
                            }
                          }
                        }
                      }
                      frame #2 {
                        n65 = property on="Setpoint\n START\n2" class="Bool"("Blinking"=FALSE) -> ()  [unwired: 2 in, 2 out]
                      }
                    }
                    n66 = Not(x="Setpoint\n START\n2") -> (.not. x?=w494:bool)
                    n67 = Unbundle(w489) -> ("VISA resource name out"=w488:refnum<visa-resource-name>, "error out"=w487:errorcluster)  [unwired: 2 out]
                  }
                  event "Standby": Value Change {
                    n68 = event-data() -> ()  [unwired: 1 in, 1 out]
                    n69 = flat-sequence {
                      tunnel: [w553] -> w543
                      tunnel: w543 -> [w557]
                      tunnel: w542 -> [w556]
                      tunnel: [w555] -> w540
                      tunnel: [w554] -> w541
                      frame #0 {
                        n70 = local read "Standby"() -> (w546:bool)
                        n71 = Select(t=TRUE, s=w546, f=FALSE) -> (s? t:f=w549:bool)
                        n72 = property on="Standby" class="Bool (strict)"("Blinking"=w549) -> ()  [unwired: 2 in, 2 out]
                      }
                      frame #1 {
                        n73 = local read "Standby"() -> (w551:bool)
                        n74 = Select(t="*D03", s=w551, f="*E03") -> (s? t:f=w553:string)
                      }
                      frame #2 {
                        n75 = Unbundle(w556) -> ("VISA resource name out"=w558:refnum<visa-resource-name>, "error out"=w560:errorcluster, "Delay (ms)"=w559:u32, "Write/\nRead"=w561:bool)
                        n76 = call "I3252_Comm_Interface.vi"("VISA resource name in"=w558, "error in"=w560, "Delay (ms)"=w559, "Write"=w561, "String to Write"=w557, "Read"=w561) -> ("VISA resource name out"=w554:refnum<visa-resource-name>, "error out"=w555:errorcluster)  [unwired: 2 in, 1 out]
                      }
                    }
                    n77 = Not(x="Standby") -> (.not. x?=w545:bool)
                    n78 = Unbundle(w539) -> ("VISA resource name out"=w538:refnum<visa-resource-name>, "error out"=w537:errorcluster)  [unwired: 2 out]
                  }
                  event "Standby\n2": Value Change {
                    n79 = event-data() -> ()  [unwired: 1 in, 1 out]
                    n80 = flat-sequence {
                      tunnel: [w578] -> w569
                      tunnel: w569 -> [w582]
                      tunnel: w567 -> [w581]
                      tunnel: [w580] -> w565
                      tunnel: [w579] -> w566
                      frame #0 {
                        n81 = local read "Standby\n2"() -> (w572:bool)
                        n82 = Select(t=TRUE, s=w572, f=FALSE) -> (s? t:f=w571:bool)
                        n83 = property on="Standby\n2" class="Bool (strict)"("Blinking"=w571) -> ()  [unwired: 2 in, 2 out]
                      }
                      frame #1 {
                        n84 = local read "Standby\n2"() -> (w576:bool)
                        n85 = Select(t="*D03", s=w576, f="*E03") -> (s? t:f=w578:string)
                      }
                      frame #2 {
                        n86 = Unbundle(w581) -> ("VISA resource name out"=w583:refnum<visa-resource-name>, "error out"=w585:errorcluster, "Delay (ms) 2"=w584:u32, "Write/\nRead \n\n2"=w586:bool)
                        n87 = call "I3252_Comm_Interface.vi"("VISA resource name in"=w583, "error in"=w585, "Delay (ms)"=w584, "Write"=w586, "String to Write"=w582, "Read"=w586) -> ("VISA resource name out"=w579:refnum<visa-resource-name>, "error out"=w580:errorcluster)  [unwired: 2 in, 1 out]
                      }
                    }
                    n88 = Not(x="Standby\n2") -> (.not. x?=w570:bool)
                    n89 = Unbundle(w564) -> ("VISA resource name out"=w563:refnum<visa-resource-name>, "error out"=w562:errorcluster)  [unwired: 2 out]
                  }
                  event "Set Command": Value Change {
                    n90 = event-data() -> ()  [unwired: 1 in, 1 out]
                    n91 = stacked-sequence {
                      tunnel: w592 -> [_ w599 _]
                      tunnel: [_ w598 _] -> w591
                      tunnel: [_ w597 _] -> w590
                      frame #0 {
                        n92 = property on="Set Command" class="Bool"("Blinking"=TRUE) -> ()  [unwired: 2 in, 2 out]
                        n93 = property on="ON" class="Bool (strict)"("Blinking"=FALSE) -> ()  [unwired: 2 in, 2 out]
                      }
                      frame #1 {
                        n94 = flat-sequence {
                          tunnel: [w604] -> w601
                          tunnel: [w607] -> w600
                          tunnel: w601 -> [w608]
                          tunnel: w599 -> [w609]
                          tunnel: [w606] -> w598
                          tunnel: [w605] -> w597
                          tunnel: w600 -> [w614]
                          frame #0 {
                            n95 = Concatenate Strings("*", "Command input") -> (w604:string)
                          }
                          frame #1 {
                            n96 = Unbundle(w609) -> ("VISA resource name out"=w613:refnum<visa-resource-name>, "error out"=w611:errorcluster, "Delay (ms)"=w612:u32, "Write/\nRead"=w610:bool)
                            n97 = call "I3252_Comm_Interface.vi"("VISA resource name in"=w613, "error in"=w611, "Delay (ms)"=w612, "Write"=w610, "String to Write"=w608, "Read"=w610) -> ("VISA resource name out"=w606:refnum<visa-resource-name>, "error out"=w605:errorcluster, "Read String"=w607:string)  [unwired: 2 in]
                          }
                          frame #2 {
                            "Command output" <- w614
                          }
                        }
                      }
                      frame #2 {
                        n98 = property on="Set Command" class="Bool"("Blinking"=FALSE) -> ()  [unwired: 2 in, 2 out]
                      }
                    }
                    n99 = Not(x="Set Command") -> (.not. x?=w594:bool)
                    n100 = Unbundle(w589) -> ("VISA resource name out"=w588:refnum<visa-resource-name>, "error out"=w587:errorcluster)  [unwired: 2 out]
                  }
                  event "Set Command\n\n 2": Value Change {
                    n101 = event-data() -> ()  [unwired: 1 in, 1 out]
                    n102 = stacked-sequence {
                      tunnel: w621 -> [_ w628 _]
                      tunnel: [_ w627 _] -> w619
                      tunnel: [_ w626 _] -> w618
                      frame #0 {
                        n103 = property on="Set Command\n\n 2" class="Bool"("Blinking"=TRUE) -> ()  [unwired: 2 in, 2 out]
                        n104 = property on="ON 2" class="Bool (strict)"("Blinking"=FALSE) -> ()  [unwired: 2 in, 2 out]
                      }
                      frame #1 {
                        n105 = flat-sequence {
                          tunnel: [w633] -> w630
                          tunnel: [w636] -> w629
                          tunnel: w630 -> [w637]
                          tunnel: w628 -> [w638]
                          tunnel: [w635] -> w627
                          tunnel: [w634] -> w626
                          tunnel: w629 -> [w643]
                          frame #0 {
                            n106 = Concatenate Strings("*", "Command input 2") -> (w633:string)
                          }
                          frame #1 {
                            n107 = Unbundle(w638) -> ("VISA resource name out"=w642:refnum<visa-resource-name>, "error out"=w640:errorcluster, "Delay (ms) 2"=w641:u32, "Write/\nRead \n\n2"=w639:bool)
                            n108 = call "I3252_Comm_Interface.vi"("VISA resource name in"=w642, "error in"=w640, "Delay (ms)"=w641, "Write"=w639, "String to Write"=w637, "Read"=w639) -> ("VISA resource name out"=w635:refnum<visa-resource-name>, "error out"=w634:errorcluster, "Read String"=w636:string)  [unwired: 2 in]
                          }
                          frame #2 {
                            "Command output 2" <- w643
                          }
                        }
                      }
                      frame #2 {
                        n109 = property on="Set Command\n\n 2" class="Bool"("Blinking"=FALSE) -> ()  [unwired: 2 in, 2 out]
                      }
                    }
                    n110 = Not(x="Set Command\n\n 2") -> (.not. x?=w623:bool)
                    n111 = Unbundle(w620) -> ("VISA resource name out"=w617:refnum<visa-resource-name>, "error out"=w616:errorcluster)  [unwired: 2 out]
                  }
                  event "Reset\nSTOP": Value Change {
                    n112 = event-data() -> ()  [unwired: 1 in, 1 out]
                    n113 = stacked-sequence {
                      tunnel: [_ w659 _] -> w649
                      tunnel: [_ w658 _] -> w650
                      tunnel: w648 -> [_ w656 _]
                      frame #0 {
                        n114 = property on="Reset\nSTOP" class="Bool"("Blinking"=TRUE) -> ()  [unwired: 2 in, 2 out]
                        n115 = property on="ON" class="Bool (strict)"("Blinking"=FALSE) -> ()  [unwired: 2 in, 2 out]
                      }
                      frame #1 {
                        n116 = for {
                          N: 2 -> [_]
                          tunnel: [w665] -> w659
                          tunnel: [w664] -> w658
                          tunnel: w656 -> [w663]
                          i -> [w661]
                          n117 = flat-sequence {
                            tunnel: w661 -> [w667]
                            tunnel: [w666] -> w662
                            tunnel: [w672] -> w665
                            tunnel: [w673] -> w664
                            tunnel: w663 -> [w674]
                            tunnel: w662 -> [w671]
                            tunnel: [w670] -> w660
                            tunnel: w661 -> [w680]
                            tunnel: w660 -> [w679]
                            frame #0 {
                              n118 = case shown="0, Default" w667 {
                                tunnel: ["*Z02" "*G01"] -> w666
                                frame 0, Default {
                                }
                                frame 1 {
                                }
                              }
                            }
                            frame #1 {
                              n119 = Unbundle(w674) -> ("VISA resource name out"=w675:refnum<visa-resource-name>, "error out"=w677:errorcluster, "Delay (ms)"=w676:u32, "Write/\nRead"=w678:bool)
                              n120 = call "I3252_Comm_Interface.vi"("VISA resource name in"=w675, "error in"=w677, "Delay (ms)"=w676, "Write"=w678, "String to Write"=w671, "Read"=w678) -> ("VISA resource name out"=w673:refnum<visa-resource-name>, "error out"=w672:errorcluster, "Read String"=w670:string)  [unwired: 2 in]
                            }
                            frame #2 {
                              n121 = case shown="0, Default" w680 {
                                tunnel: w679 -> [_ w682]
                                frame 0, Default {
                                }
                                frame 1 {
                                n122 = call "I3252_Edit_Setpoint.vi"("Read String"=w682) -> ("Setpoint is"=w681:dbl)
                                n123 = local write "SP 1 is (°C)"(w681) -> ()
                                }
                              }
                            }
                          }
                        }
                        n124 = Wait (ms)(milliseconds to wait=u32 4000) -> ()  [unwired: 1 out]
                      }
                      frame #2 {
                        n125 = property on="Reset\nSTOP" class="Bool"("Blinking"=FALSE) -> ()  [unwired: 2 in, 2 out]
                      }
                    }
                    n126 = Not(x="Reset\nSTOP") -> (.not. x?=w652:bool)
                    n127 = Unbundle(w645) -> ("VISA resource name out"=w647:refnum<visa-resource-name>, "error out"=w646:errorcluster)  [unwired: 2 out]
                  }
                  event "Reset\nSTOP 2": Value Change {
                    n128 = event-data() -> ()  [unwired: 1 in, 1 out]
                    n129 = stacked-sequence {
                      tunnel: [_ w698 _] -> w687
                      tunnel: [_ w697 _] -> w688
                      tunnel: w689 -> [_ w695 _]
                      frame #0 {
                        n130 = property on="Reset\nSTOP 2" class="Bool"("Blinking"=TRUE) -> ()  [unwired: 2 in, 2 out]
                        n131 = property on="ON 2" class="Bool (strict)"("Blinking"=FALSE) -> ()  [unwired: 2 in, 2 out]
                      }
                      frame #1 {
                        n132 = for {
                          N: 2 -> [_]
                          tunnel: [w704] -> w698
                          tunnel: [w703] -> w697
                          tunnel: w695 -> [w702]
                          i -> [w700]
                          n133 = flat-sequence {
                            tunnel: w700 -> [w706]
                            tunnel: [w705] -> w701
                            tunnel: [w711] -> w704
                            tunnel: [w712] -> w703
                            tunnel: w702 -> [w713]
                            tunnel: w701 -> [w710]
                            tunnel: [w709] -> w699
                            tunnel: w700 -> [w719]
                            tunnel: w699 -> [w718]
                            frame #0 {
                              n134 = case shown="0, Default" w706 {
                                tunnel: ["*Z02" "*G01"] -> w705
                                frame 0, Default {
                                }
                                frame 1 {
                                }
                              }
                            }
                            frame #1 {
                              n135 = Unbundle(w713) -> ("VISA resource name out"=w714:refnum<visa-resource-name>, "error out"=w716:errorcluster, "Delay (ms) 2"=w715:u32, "Write/\nRead \n\n2"=w717:bool)
                              n136 = call "I3252_Comm_Interface.vi"("VISA resource name in"=w714, "error in"=w716, "Delay (ms)"=w715, "Write"=w717, "String to Write"=w710, "Read"=w717) -> ("VISA resource name out"=w712:refnum<visa-resource-name>, "error out"=w711:errorcluster, "Read String"=w709:string)  [unwired: 2 in]
                            }
                            frame #2 {
                              n137 = case shown="1" w719 {
                                tunnel: w718 -> [_ w721]
                                frame 0, Default {
                                }
                                frame 1 {
                                n138 = call "I3252_Edit_Setpoint.vi"("Read String"=w721) -> ("Setpoint is"=w720:dbl)
                                n139 = local write "SP 2 is (°C)"(w720) -> ()
                                }
                              }
                            }
                          }
                        }
                        n140 = Wait (ms)(milliseconds to wait=u32 4000) -> ()  [unwired: 1 out]
                      }
                      frame #2 {
                        n141 = property on="Reset\nSTOP 2" class="Bool"("Blinking"=FALSE) -> ()  [unwired: 2 in, 2 out]
                      }
                    }
                    n142 = Not(x="Reset\nSTOP 2") -> (.not. x?=w691:bool)
                    n143 = Unbundle(w686) -> ("VISA resource name out"=w685:refnum<visa-resource-name>, "error out"=w684:errorcluster)  [unwired: 2 out]
                  }
                  event "Auto Tune": Value Change {
                    n144 = event-data() -> ()  [unwired: 1 in, 1 out]
                    n145 = stacked-sequence {
                      tunnel: w728 -> [_ w735 w780]
                      tunnel: [_ w734 _] -> w727
                      tunnel: [_ w733 _] -> w726
                      frame #0 {
                        n146 = property on="Auto Tune" class="Bool"("Blinking"=TRUE) -> ()  [unwired: 2 in, 2 out]
                        n147 = property on="ON" class="Bool (strict)"("Blinking"=FALSE) -> ()  [unwired: 2 in, 2 out]
                      }
                      frame #1 {
                        n148 = for {
                          N: 4 -> [_]
                          tunnel: [w740] -> w733
                          tunnel: [w739] -> w734
                          tunnel: w735 -> [w738]
                          i -> [w743]
                          n149 = flat-sequence {
                            tunnel: w743 -> [w745]
                            tunnel: [w744] -> w741
                            tunnel: w741 -> [w760]
                            tunnel: [w759] -> w742
                            tunnel: [w762] -> w740
                            tunnel: [w761] -> w739
                            tunnel: w738 -> [w758]
                            tunnel: w743 -> [w768]
                            tunnel: w742 -> [w767]
                            frame #0 {
                              n150 = case shown="0, Default" w745 {
                                tunnel: ["*V01" w748 "*W0C35" "*Z02"] -> w744
                                frame 0, Default {
                                }
                                frame 1 {
                                n151 = local read "(°C)"() -> (w747:dbl)
                                n152 = Add(x=20.0, y=w747) -> (x+y=w754:dbl)
                                n153 = Multiply(x=10.0, y=w754) -> (x*y=w751:dbl)
                                n154 = Number To Hexadecimal String(1:i16 5 ("width (-)"), 2:w751) -> (0:w750:string)
                                n155 = Concatenate Strings("*W012", w750) -> (w748:string)
                                }
                                frame 2 {
                                # "35 hex = \n00110101 bin"
                                }
                                frame 3 {
                                }
                              }
                            }
                            frame #1 {
                              n156 = Unbundle(w758) -> ("VISA resource name out"=w766:refnum<visa-resource-name>, "error out"=w764:errorcluster, "Delay (ms)"=w765:u32, "Write/\nRead"=w763:bool)
                              n157 = call "I3252_Comm_Interface.vi"("VISA resource name in"=w766, "error in"=w764, "Delay (ms)"=w765, "Write"=w763, "String to Write"=w760, "Read"=w763) -> ("VISA resource name out"=w762:refnum<visa-resource-name>, "error out"=w761:errorcluster, "Read String"=w759:string)  [unwired: 2 in]
                            }
                            frame #2 {
                              n158 = case shown="0, Default" w768 {
                                tunnel: w767 -> [w770]
                                frame 0, Default {
                                n159 = call <vilib>:"Space Constant.vi"() -> ("String"=w773:string)
                                n160 = Search/Split String(string=w770, search string/char (-)=w773) -> (match + rest of string=w772:string)  [unwired: 1 in, 2 out]
                                n161 = Fract/Exp String To Number(use system decimal point (T)=FALSE, string=w772) -> (number=w769:dbl)  [unwired: 2 in, 1 out]
                                n162 = local write "(°C)"(w769) -> ()
                                }
                              }
                            }
                          }
                        }
                        n163 = Wait (ms)(milliseconds to wait=u32 45000) -> ()  [unwired: 1 out]
                      }
                      frame #2 {
                        n164 = Unbundle(w780) -> ("VISA resource name out"=w779:refnum<visa-resource-name>, "error out"=w777:errorcluster, "Delay (ms)"=w778:u32, "Write/\nRead"=w776:bool)
                        n165 = property on="Auto Tune" class="Bool"("Blinking"=FALSE) -> ()  [unwired: 2 in, 2 out]
                        n166 = call "I3252_Comm_Interface.vi"("VISA resource name in"=w779, "error in"=w777, "Delay (ms)"=w778, "Write"=w776, "String to Write"="*W01200000", "Read"=w776) -> ()  [unwired: 2 in, 3 out]
                      }
                    }
                    n167 = Not(x="Auto Tune") -> (.not. x?=w729:bool)
                    n168 = Unbundle(w725) -> ("VISA resource name out"=w724:refnum<visa-resource-name>, "error out"=w723:errorcluster)  [unwired: 2 out]
                  }
                  event "Auto Tune 2": Value Change {
                    n169 = event-data() -> ()  [unwired: 1 in, 1 out]
                    n170 = stacked-sequence {
                      tunnel: w781 -> [_ w793 w838]
                      tunnel: [_ w792 _] -> w785
                      tunnel: [_ w791 _] -> w786
                      frame #0 {
                        n171 = property on="Auto Tune 2" class="Bool"("Blinking"=TRUE) -> ()  [unwired: 2 in, 2 out]
                        n172 = property on="ON" class="Bool (strict)"("Blinking"=FALSE) -> ()  [unwired: 2 in, 2 out]
                      }
                      frame #1 {
                        n173 = for {
                          N: 4 -> [_]
                          tunnel: [w798] -> w791
                          tunnel: [w797] -> w792
                          tunnel: w793 -> [w796]
                          i -> [w801]
                          n174 = flat-sequence {
                            tunnel: w801 -> [w803]
                            tunnel: [w802] -> w799
                            tunnel: w799 -> [w818]
                            tunnel: [w817] -> w800
                            tunnel: [w820] -> w798
                            tunnel: [w819] -> w797
                            tunnel: w796 -> [w816]
                            tunnel: w801 -> [w826]
                            tunnel: w800 -> [w825]
                            frame #0 {
                              n175 = case shown="1" w803 {
                                tunnel: ["*V01" w806 "*W0C35" "*Z02"] -> w802
                                frame 0, Default {
                                }
                                frame 1 {
                                n176 = local read "(°C) 2"() -> (w805:dbl)
                                n177 = Add(x=20.0, y=w805) -> (x+y=w812:dbl)
                                n178 = Multiply(x=10.0, y=w812) -> (x*y=w809:dbl)
                                n179 = Number To Hexadecimal String(1:i16 5 ("width (-)"), 2:w809) -> (0:w808:string)
                                n180 = Concatenate Strings("*W012", w808) -> (w806:string)
                                }
                                frame 2 {
                                # "35 hex = \n00110101 bin"
                                }
                                frame 3 {
                                }
                              }
                            }
                            frame #1 {
                              n181 = Unbundle(w816) -> ("VISA resource name out"=w824:refnum<visa-resource-name>, "error out"=w822:errorcluster, "Delay (ms) 2"=w823:u32, "Write/\nRead \n\n2"=w821:bool)
                              n182 = call "I3252_Comm_Interface.vi"("VISA resource name in"=w824, "error in"=w822, "Delay (ms)"=w823, "Write"=w821, "String to Write"=w818, "Read"=w821) -> ("VISA resource name out"=w820:refnum<visa-resource-name>, "error out"=w819:errorcluster, "Read String"=w817:string)  [unwired: 2 in]
                            }
                            frame #2 {
                              n183 = case shown="0, Default" w826 {
                                tunnel: w825 -> [w828]
                                frame 0, Default {
                                n184 = call <vilib>:"Space Constant.vi"() -> ("String"=w831:string)
                                n185 = Search/Split String(string=w828, search string/char (-)=w831) -> (match + rest of string=w830:string)  [unwired: 1 in, 2 out]
                                n186 = Fract/Exp String To Number(use system decimal point (T)=FALSE, string=w830) -> (number=w827:dbl)  [unwired: 2 in, 1 out]
                                n187 = local write "(°C) 2"(w827) -> ()
                                }
                              }
                            }
                          }
                        }
                        n188 = Wait (ms)(milliseconds to wait=u32 45000) -> ()  [unwired: 1 out]
                      }
                      frame #2 {
                        n189 = Unbundle(w838) -> ("VISA resource name out"=w837:refnum<visa-resource-name>, "error out"=w835:errorcluster, "Delay (ms) 2"=w836:u32, "Write/\nRead \n\n2"=w834:bool)
                        n190 = property on="Auto Tune 2" class="Bool"("Blinking"=FALSE) -> ()  [unwired: 2 in, 2 out]
                        n191 = call "I3252_Comm_Interface.vi"("VISA resource name in"=w837, "error in"=w835, "Delay (ms)"=w836, "Write"=w834, "String to Write"="*W01200000", "Read"=w834) -> ()  [unwired: 2 in, 3 out]
                      }
                    }
                    n192 = Not(x="Auto Tune 2") -> (.not. x?=w787:bool)
                    n193 = Unbundle(w782) -> ("VISA resource name out"=w784:refnum<visa-resource-name>, "error out"=w783:errorcluster)  [unwired: 2 out]
                  }
                  event "Write LOW/HI": Value Change {
                    n194 = event-data() -> ()  [unwired: 1 in, 1 out]
                    n195 = stacked-sequence {
                      tunnel: [_ w851 _] -> w844
                      tunnel: [_ w850 _] -> w843
                      tunnel: w842 -> [_ w849 _]
                      frame #0 {
                        n196 = property on="Write LOW/HI" class="Bool"("Blinking"=TRUE) -> ()  [unwired: 2 in, 2 out]
                        n197 = property on="ON" class="Bool (strict)"("Blinking"=FALSE) -> ()  [unwired: 2 in, 2 out]
                      }
                      frame #1 {
                        n198 = for {
                          N: 4 -> [_]
                          tunnel: [w855] -> w851
                          tunnel: [w854] -> w850
                          tunnel: w849 -> [w853]
                          i -> [w857]
                          n199 = flat-sequence {
                            tunnel: w857 -> [w859]
                            tunnel: [w860] -> w856
                            tunnel: w856 -> [w874]
                            tunnel: [w875] -> w858
                            tunnel: [w877] -> w855
                            tunnel: [w876] -> w854
                            tunnel: w853 -> [w873]
                            tunnel: w858 -> [w883]
                            tunnel: w857 -> [w882]
                            frame #0 {
                              n200 = case shown="0, Default" w859 {
                                tunnel: [w862 w868 "*R27" "*R28"] -> w860
                                frame 0, Default {
                                n201 = Number To Hexadecimal String(1:i16 2 ("width (-)"), 2:"% LOW Sollwert") -> (0:w863:string)
                                n202 = Concatenate Strings("*W27", w863) -> (w862:string)
                                }
                                frame 1 {
                                n203 = Number To Hexadecimal String(1:i16 2 ("width (-)"), 2:"% High Sollwert") -> (0:w869:string)
                                n204 = Concatenate Strings("*W28", w869) -> (w868:string)
                                }
                                frame 2 {
                                }
                                frame 3 {
                                }
                              }
                            }
                            frame #1 {
                              n205 = Unbundle(w873) -> ("VISA resource name out"=w881:refnum<visa-resource-name>, "error out"=w879:errorcluster, "Delay (ms)"=w880:u32, "Write/\nRead"=w878:bool)
                              n206 = call "I3252_Comm_Interface.vi"("VISA resource name in"=w881, "error in"=w879, "Delay (ms)"=w880, "Write"=w878, "String to Write"=w874, "Read"=w878) -> ("VISA resource name out"=w877:refnum<visa-resource-name>, "error out"=w876:errorcluster, "Read String"=w875:string)  [unwired: 2 in]
                            }
                            frame #2 {
                              n207 = case shown="0, Default" w882 {
                                tunnel: w883 -> [_ w887 w891]
                                frame 0, Default {
                                }
                                frame 2 {
                                n208 = String Subset(string=w887, offset (0)=3) -> (substring=w885:string)  [unwired: 1 in]
                                n209 = Hexadecimal String To Number(string=w885) -> (number=→"% LOW Istwert":u32)  [unwired: 2 in, 1 out]
                                }
                                frame 3 {
                                n210 = String Subset(string=w891, offset (0)=3) -> (substring=w889:string)  [unwired: 1 in]
                                n211 = Hexadecimal String To Number(string=w889) -> (number=→"% HIGH Istwert":u32)  [unwired: 2 in, 1 out]
                                }
                              }
                            }
                          }
                        }
                      }
                      frame #2 {
                        n212 = property on="Write LOW/HI" class="Bool"("Blinking"=FALSE) -> ()  [unwired: 2 in, 2 out]
                      }
                    }
                    n213 = Not(x="Write LOW/HI") -> (.not. x?=w846:bool)
                    n214 = Unbundle(w841) -> ("VISA resource name out"=w840:refnum<visa-resource-name>, "error out"=w839:errorcluster)  [unwired: 2 out]
                  }
                  event "Write LOW/HI 2": Value Change {
                    n215 = event-data() -> ()  [unwired: 1 in, 1 out]
                    n216 = stacked-sequence {
                      tunnel: [_ w905 _] -> w894
                      tunnel: [_ w904 _] -> w893
                      tunnel: w895 -> [_ w903 _]
                      frame #0 {
                        n217 = property on="Write LOW/HI 2" class="Bool"("Blinking"=TRUE) -> ()  [unwired: 2 in, 2 out]
                        n218 = property on="ON 2" class="Bool (strict)"("Blinking"=FALSE) -> ()  [unwired: 2 in, 2 out]
                      }
                      frame #1 {
                        n219 = for {
                          N: 4 -> [_]
                          tunnel: [w909] -> w905
                          tunnel: [w908] -> w904
                          tunnel: w903 -> [w907]
                          i -> [w911]
                          n220 = flat-sequence {
                            tunnel: w911 -> [w913]
                            tunnel: [w914] -> w910
                            tunnel: w910 -> [w928]
                            tunnel: [w929] -> w912
                            tunnel: [w931] -> w909
                            tunnel: [w930] -> w908
                            tunnel: w907 -> [w927]
                            tunnel: w912 -> [w937]
                            tunnel: w911 -> [w936]
                            frame #0 {
                              n221 = case shown="0, Default" w913 {
                                tunnel: [w917 w922 "*R27" "*R28"] -> w914
                                frame 0, Default {
                                n222 = Number To Hexadecimal String(1:i16 2 ("width (-)"), 2:"% LOW Sollwert 2") -> (0:w918:string)
                                n223 = Concatenate Strings("*W27", w918) -> (w917:string)
                                }
                                frame 1 {
                                n224 = Number To Hexadecimal String(1:i16 2 ("width (-)"), 2:"% High Sollwert 2") -> (0:w923:string)
                                n225 = Concatenate Strings("*W28", w923) -> (w922:string)
                                }
                                frame 2 {
                                }
                                frame 3 {
                                }
                              }
                            }
                            frame #1 {
                              n226 = Unbundle(w927) -> ("VISA resource name out"=w935:refnum<visa-resource-name>, "error out"=w933:errorcluster, "Delay (ms) 2"=w934:u32, "Write/\nRead \n\n2"=w932:bool)
                              n227 = call "I3252_Comm_Interface.vi"("VISA resource name in"=w935, "error in"=w933, "Delay (ms)"=w934, "Write"=w932, "String to Write"=w928, "Read"=w932) -> ("VISA resource name out"=w931:refnum<visa-resource-name>, "error out"=w930:errorcluster, "Read String"=w929:string)  [unwired: 2 in]
                            }
                            frame #2 {
                              n228 = case shown="3" w936 {
                                tunnel: w937 -> [_ w941 w945]
                                frame 0, Default {
                                }
                                frame 2 {
                                n229 = String Subset(string=w941, offset (0)=3) -> (substring=w939:string)  [unwired: 1 in]
                                n230 = Hexadecimal String To Number(string=w939) -> (number=→"% LOW Istwert 2":u32)  [unwired: 2 in, 1 out]
                                }
                                frame 3 {
                                n231 = String Subset(string=w945, offset (0)=3) -> (substring=w943:string)  [unwired: 1 in]
                                n232 = Hexadecimal String To Number(string=w943) -> (number=→"% HIGH Istwert 2":u32)  [unwired: 2 in, 1 out]
                                }
                              }
                            }
                          }
                        }
                      }
                      frame #2 {
                        n233 = property on="Write LOW/HI 2" class="Bool"("Blinking"=FALSE) -> ()  [unwired: 2 in, 2 out]
                      }
                    }
                    n234 = Not(x="Write LOW/HI 2") -> (.not. x?=w900:bool)
                    n235 = Unbundle(w898) -> ("VISA resource name out"=w897:refnum<visa-resource-name>, "error out"=w896:errorcluster)  [unwired: 2 out]
                  }
                  event "Set PID": Value Change {
                    n236 = event-data() -> ()  [unwired: 1 in, 1 out]
                    n237 = stacked-sequence {
                      tunnel: w952 -> [_ w959 _]
                      tunnel: [_ w958 _] -> w951
                      tunnel: [_ w957 _] -> w950
                      frame #0 {
                        n238 = property on="Set PID" class="Bool"("Blinking"=TRUE) -> ()  [unwired: 2 in, 2 out]
                        n239 = property on="ON" class="Bool (strict)"("Blinking"=FALSE) -> ()  [unwired: 2 in, 2 out]
                      }
                      frame #1 {
                        n240 = for {
                          N: 6 -> [_]
                          tunnel: w959 -> [w963]
                          tunnel: [w962] -> w958
                          tunnel: [w961] -> w957
                          i -> [w965]
                          n241 = flat-sequence {
                            tunnel: w965 -> [w967]
                            tunnel: [w968] -> w964
                            tunnel: w964 -> [w1009]
                            tunnel: [w1005] -> w966
                            tunnel: w963 -> [w1008]
                            tunnel: [w1007] -> w961
                            tunnel: [w1006] -> w962
                            tunnel: w966 -> [w1015]
                            tunnel: w965 -> [w1014]
                            frame #0 {
                              n242 = case shown="2" w967 {
                                tunnel: [w975 w983 w991 w993 w997 w1001] -> w968
                                frame 0, Default {
                                n243 = local read "RAM"() -> (w969:bool)
                                n244 = Number To Hexadecimal String(1:i16 4 ("width (-)"), 2:"P (PB1) Sollwert") -> (0:w976:string)
                                n245 = Select(t="*P17", s=w969, f="*W17") -> (s? t:f=w970:string)
                                n246 = Concatenate Strings(w970, w976) -> (w975:string)
                                }
                                frame 1 {
                                n247 = local read "RAM"() -> (w977:bool)
                                n248 = Number To Hexadecimal String(1:i16 4 ("width (-)"), 2:"I ( Reset1) Sollwert") -> (0:w984:string)
                                n249 = Select(t="*P18", s=w977, f="*W18") -> (s? t:f=w979:string)
                                n250 = Concatenate Strings(w979, w984) -> (w983:string)
                                }
                                frame 2 {
                                n251 = local read "RAM"() -> (w986:bool)
                                n252 = Number To Hexadecimal String(1:i16 4 ("width (-)"), 2:"D (Rate) Sollwert") -> (0:w992:string)
                                n253 = Select(t="*P19", s=w986, f="*W19") -> (s? t:f=w987:string)
                                n254 = Concatenate Strings(w987, w992) -> (w991:string)
                                }
                                frame 3 {
                                n255 = local read "RAM"() -> (w996:bool)
                                n256 = Select(t="*G17", s=w996, f="*R17") -> (s? t:f=w993:string)
                                }
                                frame 4 {
                                n257 = local read "RAM"() -> (w1000:bool)
                                n258 = Select(t="*G18", s=w1000, f="*R18") -> (s? t:f=w997:string)
                                }
                                frame 5 {
                                n259 = local read "RAM"() -> (w1004:bool)
                                n260 = Select(t="*G19", s=w1004, f="*R19") -> (s? t:f=w1001:string)
                                }
                              }
                            }
                            frame #1 {
                              n261 = Unbundle(w1008) -> ("VISA resource name out"=w1013:refnum<visa-resource-name>, "error out"=w1011:errorcluster, "Delay (ms)"=w1012:u32, "Write/\nRead"=w1010:bool)
                              n262 = call "I3252_Comm_Interface.vi"("VISA resource name in"=w1013, "error in"=w1011, "Delay (ms)"=w1012, "Write"=w1010, "String to Write"=w1009, "Read"=w1010) -> ("VISA resource name out"=w1006:refnum<visa-resource-name>, "error out"=w1007:errorcluster, "Read String"=w1005:string)  [unwired: 2 in]
                            }
                            frame #2 {
                              n263 = case shown="4" w1014 {
                                tunnel: w1015 -> [_ w1019 w1023 w1027]
                                frame 0, Default {
                                }
                                frame 3 {
                                n264 = String Subset(string=w1019, offset (0)=3) -> (substring=w1017:string)  [unwired: 1 in]
                                n265 = Hexadecimal String To Number(string=w1017) -> (number=→"P (PB1) Istwert":u32)  [unwired: 2 in, 1 out]
                                }
                                frame 4 {
                                n266 = String Subset(string=w1023, offset (0)=3) -> (substring=w1021:string)  [unwired: 1 in]
                                n267 = Hexadecimal String To Number(string=w1021) -> (number=→"I ( Reset1) Istwert":u32)  [unwired: 2 in, 1 out]
                                }
                                frame 5 {
                                n268 = String Subset(string=w1027, offset (0)=3) -> (substring=w1025:string)  [unwired: 1 in]
                                n269 = Hexadecimal String To Number(string=w1025) -> (number=→"D (Rate) IstWert":u32)  [unwired: 2 in, 1 out]
                                }
                              }
                            }
                          }
                        }
                      }
                      frame #2 {
                        n270 = property on="Set PID" class="Bool"("Blinking"=FALSE) -> ()  [unwired: 2 in, 2 out]
                      }
                    }
                    n271 = Not(x="Set PID") -> (.not. x?=w954:bool)
                    n272 = Unbundle(w949) -> ("VISA resource name out"=w948:refnum<visa-resource-name>, "error out"=w947:errorcluster)  [unwired: 2 out]
                  }
                  event "Set PID 2": Value Change {
                    n273 = event-data() -> ()  [unwired: 1 in, 1 out]
                    n274 = stacked-sequence {
                      tunnel: w1029 -> [_ w1041 _]
                      tunnel: [_ w1040 _] -> w1031
                      tunnel: [_ w1039 _] -> w1030
                      frame #0 {
                        n275 = property on="Set PID 2" class="Bool"("Blinking"=TRUE) -> ()  [unwired: 2 in, 2 out]
                        n276 = property on="ON 2" class="Bool (strict)"("Blinking"=FALSE) -> ()  [unwired: 2 in, 2 out]
                      }
                      frame #1 {
                        n277 = for {
                          N: 6 -> [_]
                          tunnel: w1041 -> [w1045]
                          tunnel: [w1044] -> w1040
                          tunnel: [w1043] -> w1039
                          i -> [w1047]
                          n278 = flat-sequence {
                            tunnel: w1047 -> [w1049]
                            tunnel: [w1050] -> w1046
                            tunnel: w1046 -> [w1091]
                            tunnel: [w1087] -> w1048
                            tunnel: w1045 -> [w1090]
                            tunnel: [w1089] -> w1043
                            tunnel: [w1088] -> w1044
                            tunnel: w1048 -> [w1097]
                            tunnel: w1047 -> [w1096]
                            frame #0 {
                              n279 = case shown="0, Default" w1049 {
                                tunnel: [w1057 w1065 w1073 w1075 w1079 w1083] -> w1050
                                frame 0, Default {
                                n280 = local read "RAM 2"() -> (w1052:bool)
                                n281 = Number To Hexadecimal String(1:i16 4 ("width (-)"), 2:"P (PB1) Sollwert 2") -> (0:w1058:string)
                                n282 = Select(t="*P17", s=w1052, f="*W17") -> (s? t:f=w1053:string)
                                n283 = Concatenate Strings(w1053, w1058) -> (w1057:string)
                                }
                                frame 1 {
                                n284 = local read "RAM 2"() -> (w1060:bool)
                                n285 = Number To Hexadecimal String(1:i16 4 ("width (-)"), 2:"I ( Reset1) Sollwert 2") -> (0:w1066:string)
                                n286 = Select(t="*P18", s=w1060, f="*W18") -> (s? t:f=w1061:string)
                                n287 = Concatenate Strings(w1061, w1066) -> (w1065:string)
                                }
                                frame 2 {
                                n288 = local read "RAM 2"() -> (w1068:bool)
                                n289 = Number To Hexadecimal String(1:i16 4 ("width (-)"), 2:"D (Rate) Sollwert 2") -> (0:w1074:string)
                                n290 = Select(t="*P19", s=w1068, f="*W19") -> (s? t:f=w1069:string)
                                n291 = Concatenate Strings(w1069, w1074) -> (w1073:string)
                                }
                                frame 3 {
                                n292 = local read "RAM"() -> (w1078:bool)
                                n293 = Select(t="*G17", s=w1078, f="*R17") -> (s? t:f=w1075:string)
                                }
                                frame 4 {
                                n294 = local read "RAM"() -> (w1082:bool)
                                n295 = Select(t="*G18", s=w1082, f="*R18") -> (s? t:f=w1079:string)
                                }
                                frame 5 {
                                n296 = local read "RAM"() -> (w1086:bool)
                                n297 = Select(t="*G19", s=w1086, f="*R19") -> (s? t:f=w1083:string)
                                }
                              }
                            }
                            frame #1 {
                              n298 = Unbundle(w1090) -> ("VISA resource name out"=w1095:refnum<visa-resource-name>, "error out"=w1093:errorcluster, "Delay (ms) 2"=w1094:u32, "Write/\nRead \n\n2"=w1092:bool)
                              n299 = call "I3252_Comm_Interface.vi"("VISA resource name in"=w1095, "error in"=w1093, "Delay (ms)"=w1094, "Write"=w1092, "String to Write"=w1091, "Read"=w1092) -> ("VISA resource name out"=w1088:refnum<visa-resource-name>, "error out"=w1089:errorcluster, "Read String"=w1087:string)  [unwired: 2 in]
                            }
                            frame #2 {
                              n300 = case shown="0, Default" w1096 {
                                tunnel: w1097 -> [_ w1101 w1105 w1109]
                                frame 0, Default {
                                }
                                frame 3 {
                                n301 = String Subset(string=w1101, offset (0)=3) -> (substring=w1099:string)  [unwired: 1 in]
                                n302 = Hexadecimal String To Number(string=w1099) -> (number=→"P (PB1) Istwert 2":u32)  [unwired: 2 in, 1 out]
                                }
                                frame 4 {
                                n303 = String Subset(string=w1105, offset (0)=3) -> (substring=w1103:string)  [unwired: 1 in]
                                n304 = Hexadecimal String To Number(string=w1103) -> (number=→"I ( Reset1) Istwert 2":u32)  [unwired: 2 in, 1 out]
                                }
                                frame 5 {
                                n305 = String Subset(string=w1109, offset (0)=3) -> (substring=w1107:string)  [unwired: 1 in]
                                n306 = Hexadecimal String To Number(string=w1107) -> (number=→"D (Rate) IstWert 2":u32)  [unwired: 2 in, 1 out]
                                }
                              }
                            }
                          }
                        }
                      }
                      frame #2 {
                        n307 = property on="Set PID 2" class="Bool"("Blinking"=FALSE) -> ()  [unwired: 2 in, 2 out]
                      }
                    }
                    n308 = Not(x="Set PID 2") -> (.not. x?=w1036:bool)
                    n309 = Unbundle(w1034) -> ("VISA resource name out"=w1033:refnum<visa-resource-name>, "error out"=w1032:errorcluster)  [unwired: 2 out]
                  }
                  event "Get Values": Value Change {
                    n310 = event-data() -> ()  [unwired: 1 in, 1 out]
                    n311 = stacked-sequence {
                      tunnel: w1116 -> [_ w1123 _]
                      tunnel: [_ w1122 _] -> w1115
                      tunnel: [_ w1121 _] -> w1114
                      frame #0 {
                        n312 = property on="Get Values" class="Bool"("Blinking"=TRUE) -> ()  [unwired: 2 in, 2 out]
                        n313 = property on="ON" class="Bool (strict)"("Blinking"=FALSE) -> ()  [unwired: 2 in, 2 out]
                      }
                      frame #1 {
                        n314 = for {
                          N: 6 -> [_]
                          tunnel: w1123 -> [w1127]
                          tunnel: [w1126] -> w1122
                          tunnel: [w1125] -> w1121
                          i -> [w1129]
                          n315 = flat-sequence {
                            tunnel: w1129 -> [w1131]
                            tunnel: [w1132] -> w1128
                            tunnel: w1128 -> [w1154]
                            tunnel: [w1155] -> w1130
                            tunnel: w1127 -> [w1153]
                            tunnel: [w1152] -> w1125
                            tunnel: [w1151] -> w1126
                            tunnel: w1130 -> [w1161]
                            tunnel: w1129 -> [w1160]
                            frame #0 {
                              n316 = case shown="0, Default" w1131 {
                                tunnel: [w1135 w1139 w1143 "*R27" "*R28" w1149] -> w1132
                                frame 0, Default {
                                n317 = local read "RAM"() -> (w1136:bool)
                                n318 = Select(t="*G17", s=w1136, f="*R17") -> (s? t:f=w1135:string)
                                }
                                frame 1 {
                                n319 = local read "RAM"() -> (w1140:bool)
                                n320 = Select(t="*G18", s=w1140, f="*R18") -> (s? t:f=w1139:string)
                                }
                                frame 2 {
                                n321 = local read "RAM"() -> (w1144:bool)
                                n322 = Select(t="*G19", s=w1144, f="*R19") -> (s? t:f=w1143:string)
                                }
                                frame 3 {
                                }
                                frame 4 {
                                }
                                frame 5 {
                                n323 = local read "RAM"() -> (w1150:bool)
                                n324 = Select(t="*G01", s=w1150, f="*R01") -> (s? t:f=w1149:string)
                                }
                              }
                            }
                            frame #1 {
                              n325 = Unbundle(w1153) -> ("VISA resource name out"=w1159:refnum<visa-resource-name>, "error out"=w1157:errorcluster, "Delay (ms)"=w1158:u32, "Write/\nRead"=w1156:bool)
                              n326 = call "I3252_Comm_Interface.vi"("VISA resource name in"=w1159, "error in"=w1157, "Delay (ms)"=w1158, "Write"=w1156, "String to Write"=w1154, "Read"=w1156) -> ("VISA resource name out"=w1151:refnum<visa-resource-name>, "error out"=w1152:errorcluster, "Read String"=w1155:string)  [unwired: 2 in]
                            }
                            frame #2 {
                              n327 = case shown="1" w1160 {
                                tunnel: w1161 -> [w1163 w1167 w1171 w1175 w1179 w1183]
                                frame 0, Default {
                                n328 = String Subset(string=w1163, offset (0)=3) -> (substring=w1164:string)  [unwired: 1 in]
                                n329 = Hexadecimal String To Number(string=w1164) -> (number=w1162:u32)  [unwired: 2 in, 1 out]
                                n330 = local write "P (PB1) Sollwert"(w1162) -> ()
                                n331 = local write "P (PB1) Istwert"(w1162) -> ()
                                }
                                frame 1 {
                                n332 = String Subset(string=w1167, offset (0)=3) -> (substring=w1168:string)  [unwired: 1 in]
                                n333 = Hexadecimal String To Number(string=w1168) -> (number=w1166:u32)  [unwired: 2 in, 1 out]
                                n334 = local write "I ( Reset1) Sollwert"(w1166) -> ()
                                n335 = local write "I ( Reset1) Istwert"(w1166) -> ()
                                }
                                frame 2 {
                                n336 = String Subset(string=w1171, offset (0)=3) -> (substring=w1172:string)  [unwired: 1 in]
                                n337 = Hexadecimal String To Number(string=w1172) -> (number=w1170:u32)  [unwired: 2 in, 1 out]
                                n338 = local write "D (Rate) Sollwert"(w1170) -> ()
                                n339 = local write "D (Rate) IstWert"(w1170) -> ()
                                }
                                frame 3 {
                                n340 = String Subset(string=w1175, offset (0)=3) -> (substring=w1176:string)  [unwired: 1 in]
                                n341 = Hexadecimal String To Number(string=w1176) -> (number=w1174:u32)  [unwired: 2 in, 1 out]
                                n342 = local write "% LOW Istwert"(w1174) -> ()
                                n343 = local write "% LOW Sollwert"(w1174) -> ()
                                }
                                frame 4 {
                                n344 = String Subset(string=w1179, offset (0)=3) -> (substring=w1180:string)  [unwired: 1 in]
                                n345 = Hexadecimal String To Number(string=w1180) -> (number=w1178:u32)  [unwired: 2 in, 1 out]
                                n346 = local write "% High Sollwert"(w1178) -> ()
                                n347 = local write "% HIGH Istwert"(w1178) -> ()
                                }
                                frame 5 {
                                n348 = call "I3252_Edit_Setpoint.vi"("Read String"=w1183) -> ("Setpoint is"=w1182:dbl)
                                n349 = local write "SP 1 is (°C)"(w1182) -> ()
                                }
                              }
                            }
                          }
                        }
                      }
                      frame #2 {
                        n350 = property on="Get Values" class="Bool"("Blinking"=FALSE) -> ()  [unwired: 2 in, 2 out]
                      }
                    }
                    n351 = Not(x="Get Values") -> (.not. x?=w1118:bool)
                    n352 = Unbundle(w1113) -> ("VISA resource name out"=w1112:refnum<visa-resource-name>, "error out"=w1111:errorcluster)  [unwired: 2 out]
                  }
                  event "Get Values 2": Value Change {
                    n353 = event-data() -> ()  [unwired: 1 in, 1 out]
                    n354 = stacked-sequence {
                      tunnel: w1187 -> [_ w1197 _]
                      tunnel: [_ w1196 _] -> w1186
                      tunnel: [_ w1195 _] -> w1185
                      frame #0 {
                        n355 = property on="Get Values 2" class="Bool"("Blinking"=TRUE) -> ()  [unwired: 2 in, 2 out]
                        n356 = property on="ON 2" class="Bool (strict)"("Blinking"=FALSE) -> ()  [unwired: 2 in, 2 out]
                      }
                      frame #1 {
                        n357 = for {
                          N: 6 -> [_]
                          tunnel: w1197 -> [w1201]
                          tunnel: [w1200] -> w1196
                          tunnel: [w1199] -> w1195
                          i -> [w1203]
                          n358 = flat-sequence {
                            tunnel: w1203 -> [w1205]
                            tunnel: [w1206] -> w1202
                            tunnel: w1202 -> [w1228]
                            tunnel: [w1229] -> w1204
                            tunnel: w1201 -> [w1227]
                            tunnel: [w1226] -> w1199
                            tunnel: [w1225] -> w1200
                            tunnel: w1204 -> [w1235]
                            tunnel: w1203 -> [w1234]
                            frame #0 {
                              n359 = case shown="1" w1205 {
                                tunnel: [w1209 w1213 w1217 "*R27" "*R28" w1223] -> w1206
                                frame 0, Default {
                                n360 = local read "RAM 2"() -> (w1210:bool)
                                n361 = Select(t="*G17", s=w1210, f="*R17") -> (s? t:f=w1209:string)
                                }
                                frame 1 {
                                n362 = local read "RAM 2"() -> (w1214:bool)
                                n363 = Select(t="*G18", s=w1214, f="*R18") -> (s? t:f=w1213:string)
                                }
                                frame 2 {
                                n364 = local read "RAM 2"() -> (w1218:bool)
                                n365 = Select(t="*G19", s=w1218, f="*R19") -> (s? t:f=w1217:string)
                                }
                                frame 3 {
                                }
                                frame 4 {
                                }
                                frame 5 {
                                n366 = local read "RAM 2"() -> (w1224:bool)
                                n367 = Select(t="*G01", s=w1224, f="*R01") -> (s? t:f=w1223:string)
                                }
                              }
                            }
                            frame #1 {
                              n368 = Unbundle(w1227) -> ("VISA resource name out"=w1233:refnum<visa-resource-name>, "error out"=w1231:errorcluster, "Delay (ms) 2"=w1232:u32, "Write/\nRead \n\n2"=w1230:bool)
                              n369 = call "I3252_Comm_Interface.vi"("VISA resource name in"=w1233, "error in"=w1231, "Delay (ms)"=w1232, "Write"=w1230, "String to Write"=w1228, "Read"=w1230) -> ("VISA resource name out"=w1225:refnum<visa-resource-name>, "error out"=w1226:errorcluster, "Read String"=w1229:string)  [unwired: 2 in]
                            }
                            frame #2 {
                              n370 = case shown="0, Default" w1234 {
                                tunnel: w1235 -> [w1237 w1241 w1245 w1249 w1253 w1257]
                                frame 0, Default {
                                n371 = String Subset(string=w1237, offset (0)=3) -> (substring=w1238:string)  [unwired: 1 in]
                                n372 = Hexadecimal String To Number(string=w1238) -> (number=w1236:u32)  [unwired: 2 in, 1 out]
                                n373 = local write "P (PB1) Sollwert 2"(w1236) -> ()
                                n374 = local write "P (PB1) Istwert 2"(w1236) -> ()
                                }
                                frame 1 {
                                n375 = String Subset(string=w1241, offset (0)=3) -> (substring=w1242:string)  [unwired: 1 in]
                                n376 = Hexadecimal String To Number(string=w1242) -> (number=w1240:u32)  [unwired: 2 in, 1 out]
                                n377 = local write "I ( Reset1) Sollwert 2"(w1240) -> ()
                                n378 = local write "I ( Reset1) Istwert 2"(w1240) -> ()
                                }
                                frame 2 {
                                n379 = String Subset(string=w1245, offset (0)=3) -> (substring=w1246:string)  [unwired: 1 in]
                                n380 = Hexadecimal String To Number(string=w1246) -> (number=w1244:u32)  [unwired: 2 in, 1 out]
                                n381 = local write "D (Rate) Sollwert 2"(w1244) -> ()
                                n382 = local write "D (Rate) IstWert 2"(w1244) -> ()
                                }
                                frame 3 {
                                n383 = String Subset(string=w1249, offset (0)=3) -> (substring=w1250:string)  [unwired: 1 in]
                                n384 = Hexadecimal String To Number(string=w1250) -> (number=w1248:u32)  [unwired: 2 in, 1 out]
                                n385 = local write "% LOW Istwert 2"(w1248) -> ()
                                n386 = local write "% LOW Sollwert 2"(w1248) -> ()
                                }
                                frame 4 {
                                n387 = String Subset(string=w1253, offset (0)=3) -> (substring=w1254:string)  [unwired: 1 in]
                                n388 = Hexadecimal String To Number(string=w1254) -> (number=w1252:u32)  [unwired: 2 in, 1 out]
                                n389 = local write "% High Sollwert 2"(w1252) -> ()
                                n390 = local write "% HIGH Istwert 2"(w1252) -> ()
                                }
                                frame 5 {
                                n391 = call "I3252_Edit_Setpoint.vi"("Read String"=w1257) -> ("Setpoint is"=w1256:dbl)
                                n392 = local write "SP 2 is (°C)"(w1256) -> ()
                                }
                              }
                            }
                          }
                        }
                      }
                      frame #2 {
                        n393 = property on="Get Values 2" class="Bool"("Blinking"=FALSE) -> ()  [unwired: 2 in, 2 out]
                      }
                    }
                    n394 = Not(x="Get Values 2") -> (.not. x?=w1192:bool)
                    n395 = Unbundle(w1188) -> ("VISA resource name out"=w1190:refnum<visa-resource-name>, "error out"=w1189:errorcluster)  [unwired: 2 out]
                  }
                  event "RAM": Value Change {
                    n396 = event-data() -> ()  [unwired: 1 in, 1 out]
                    n397 = stacked-sequence {
                      tunnel: w1264 -> [_ w1271 _]
                      tunnel: [_ w1270 _] -> w1263
                      tunnel: [_ w1269 _] -> w1262
                      frame #0 {
                        n398 = property on="RAM" class="Bool (strict)"("Blinking"=TRUE) -> ()  [unwired: 2 in, 2 out]
                        n399 = property on="ON" class="Bool (strict)"("Blinking"=FALSE) -> ()  [unwired: 2 in, 2 out]
                      }
                      frame #1 {
                        n400 = for {
                          N: 6 -> [_]
                          tunnel: w1271 -> [w1275]
                          tunnel: [w1274] -> w1270
                          tunnel: [w1273] -> w1269
                          i -> [w1277]
                          n401 = flat-sequence {
                            tunnel: w1277 -> [w1279]
                            tunnel: [w1280] -> w1276
                            tunnel: w1276 -> [w1299]
                            tunnel: [w1300] -> w1278
                            tunnel: w1275 -> [w1303]
                            tunnel: [w1302] -> w1273
                            tunnel: [w1301] -> w1274
                            tunnel: w1278 -> [w1309]
                            tunnel: w1277 -> [w1308]
                            frame #0 {
                              n402 = case shown="3" w1279 {
                                tunnel: [w1283 w1287 w1291 "*R27" "*R28" w1297] -> w1280
                                frame 0, Default {
                                n403 = local read "RAM"() -> (w1284:bool)
                                n404 = Select(t="*G17", s=w1284, f="*R17") -> (s? t:f=w1283:string)
                                }
                                frame 1 {
                                n405 = local read "RAM"() -> (w1288:bool)
                                n406 = Select(t="*G18", s=w1288, f="*R18") -> (s? t:f=w1287:string)
                                }
                                frame 2 {
                                n407 = local read "RAM"() -> (w1292:bool)
                                n408 = Select(t="*G19", s=w1292, f="*R19") -> (s? t:f=w1291:string)
                                }
                                frame 3 {
                                }
                                frame 4 {
                                }
                                frame 5 {
                                n409 = local read "RAM"() -> (w1298:bool)
                                n410 = Select(t="*G01", s=w1298, f="*R01") -> (s? t:f=w1297:string)
                                }
                              }
                            }
                            frame #1 {
                              n411 = Unbundle(w1303) -> ("VISA resource name out"=w1307:refnum<visa-resource-name>, "error out"=w1305:errorcluster, "Delay (ms)"=w1306:u32, "Write/\nRead"=w1304:bool)
                              n412 = call "I3252_Comm_Interface.vi"("VISA resource name in"=w1307, "error in"=w1305, "Delay (ms)"=w1306, "Write"=w1304, "String to Write"=w1299, "Read"=w1304) -> ("VISA resource name out"=w1301:refnum<visa-resource-name>, "error out"=w1302:errorcluster, "Read String"=w1300:string)  [unwired: 2 in]
                            }
                            frame #2 {
                              n413 = case shown="5" w1308 {
                                tunnel: w1309 -> [w1311 w1315 w1319 w1323 w1327 w1331]
                                frame 0, Default {
                                n414 = String Subset(string=w1311, offset (0)=3) -> (substring=w1312:string)  [unwired: 1 in]
                                n415 = Hexadecimal String To Number(string=w1312) -> (number=w1310:u32)  [unwired: 2 in, 1 out]
                                n416 = local write "P (PB1) Sollwert"(w1310) -> ()
                                n417 = local write "P (PB1) Istwert"(w1310) -> ()
                                }
                                frame 1 {
                                n418 = String Subset(string=w1315, offset (0)=3) -> (substring=w1316:string)  [unwired: 1 in]
                                n419 = Hexadecimal String To Number(string=w1316) -> (number=w1314:u32)  [unwired: 2 in, 1 out]
                                n420 = local write "I ( Reset1) Sollwert"(w1314) -> ()
                                n421 = local write "I ( Reset1) Istwert"(w1314) -> ()
                                }
                                frame 2 {
                                n422 = String Subset(string=w1319, offset (0)=3) -> (substring=w1320:string)  [unwired: 1 in]
                                n423 = Hexadecimal String To Number(string=w1320) -> (number=w1318:u32)  [unwired: 2 in, 1 out]
                                n424 = local write "D (Rate) IstWert"(w1318) -> ()
                                n425 = local write "D (Rate) Sollwert"(w1318) -> ()
                                }
                                frame 3 {
                                n426 = String Subset(string=w1323, offset (0)=3) -> (substring=w1324:string)  [unwired: 1 in]
                                n427 = Hexadecimal String To Number(string=w1324) -> (number=w1322:u32)  [unwired: 2 in, 1 out]
                                n428 = local write "% LOW Istwert"(w1322) -> ()
                                n429 = local write "% LOW Sollwert"(w1322) -> ()
                                }
                                frame 4 {
                                n430 = String Subset(string=w1327, offset (0)=3) -> (substring=w1328:string)  [unwired: 1 in]
                                n431 = Hexadecimal String To Number(string=w1328) -> (number=w1326:u32)  [unwired: 2 in, 1 out]
                                n432 = local write "% HIGH Istwert"(w1326) -> ()
                                n433 = local write "% High Sollwert"(w1326) -> ()
                                }
                                frame 5 {
                                n434 = call "I3252_Edit_Setpoint.vi"("Read String"=w1331) -> ("Setpoint is"=w1330:dbl)
                                n435 = local write "SP 1 is (°C)"(w1330) -> ()
                                }
                              }
                            }
                          }
                        }
                      }
                      frame #2 {
                        n436 = property on="RAM" class="Bool (strict)"("Blinking"=FALSE) -> ()  [unwired: 2 in, 2 out]
                      }
                    }
                    n437 = Not(x="RAM") -> (.not. x?=w1266:bool)
                    n438 = Unbundle(w1261) -> ("VISA resource name out"=w1260:refnum<visa-resource-name>, "error out"=w1259:errorcluster)  [unwired: 2 out]
                  }
                  event "RAM 2": Value Change {
                    n439 = event-data() -> ()  [unwired: 1 in, 1 out]
                    n440 = stacked-sequence {
                      tunnel: w1335 -> [_ w1345 _]
                      tunnel: [_ w1344 _] -> w1334
                      tunnel: [_ w1343 _] -> w1333
                      frame #0 {
                        n441 = property on="RAM 2" class="Bool (strict)"("Blinking"=TRUE) -> ()  [unwired: 2 in, 2 out]
                        n442 = property on="ON 2" class="Bool (strict)"("Blinking"=FALSE) -> ()  [unwired: 2 in, 2 out]
                      }
                      frame #1 {
                        n443 = for {
                          N: 6 -> [_]
                          tunnel: w1345 -> [w1349]
                          tunnel: [w1348] -> w1344
                          tunnel: [w1347] -> w1343
                          i -> [w1351]
                          n444 = flat-sequence {
                            tunnel: w1351 -> [w1353]
                            tunnel: [w1354] -> w1350
                            tunnel: w1350 -> [w1373]
                            tunnel: [w1374] -> w1352
                            tunnel: w1349 -> [w1377]
                            tunnel: [w1376] -> w1347
                            tunnel: [w1375] -> w1348
                            tunnel: w1352 -> [w1383]
                            tunnel: w1351 -> [w1382]
                            frame #0 {
                              n445 = case shown="5" w1353 {
                                tunnel: [w1357 w1361 w1365 "*R27" "*R28" w1371] -> w1354
                                frame 0, Default {
                                n446 = local read "RAM 2"() -> (w1358:bool)
                                n447 = Select(t="*G17", s=w1358, f="*R17") -> (s? t:f=w1357:string)
                                }
                                frame 1 {
                                n448 = local read "RAM 2"() -> (w1362:bool)
                                n449 = Select(t="*G18", s=w1362, f="*R18") -> (s? t:f=w1361:string)
                                }
                                frame 2 {
                                n450 = local read "RAM 2"() -> (w1366:bool)
                                n451 = Select(t="*G19", s=w1366, f="*R19") -> (s? t:f=w1365:string)
                                }
                                frame 3 {
                                }
                                frame 4 {
                                }
                                frame 5 {
                                n452 = local read "RAM 2"() -> (w1372:bool)
                                n453 = Select(t="*G01", s=w1372, f="*R01") -> (s? t:f=w1371:string)
                                }
                              }
                            }
                            frame #1 {
                              n454 = Unbundle(w1377) -> ("VISA resource name out"=w1381:refnum<visa-resource-name>, "error out"=w1379:errorcluster, "Delay (ms) 2"=w1380:u32, "Write/\nRead \n\n2"=w1378:bool)
                              n455 = call "I3252_Comm_Interface.vi"("VISA resource name in"=w1381, "error in"=w1379, "Delay (ms)"=w1380, "Write"=w1378, "String to Write"=w1373, "Read"=w1378) -> ("VISA resource name out"=w1375:refnum<visa-resource-name>, "error out"=w1376:errorcluster, "Read String"=w1374:string)  [unwired: 2 in]
                            }
                            frame #2 {
                              n456 = case shown="0, Default" w1382 {
                                tunnel: w1383 -> [w1385 w1389 w1393 w1397 w1401 w1405]
                                frame 0, Default {
                                n457 = String Subset(string=w1385, offset (0)=3) -> (substring=w1386:string)  [unwired: 1 in]
                                n458 = Hexadecimal String To Number(string=w1386) -> (number=w1384:u32)  [unwired: 2 in, 1 out]
                                n459 = local write "P (PB1) Sollwert 2"(w1384) -> ()
                                n460 = local write "P (PB1) Istwert 2"(w1384) -> ()
                                }
                                frame 1 {
                                n461 = String Subset(string=w1389, offset (0)=3) -> (substring=w1390:string)  [unwired: 1 in]
                                n462 = Hexadecimal String To Number(string=w1390) -> (number=w1388:u32)  [unwired: 2 in, 1 out]
                                n463 = local write "I ( Reset1) Sollwert 2"(w1388) -> ()
                                n464 = local write "I ( Reset1) Istwert 2"(w1388) -> ()
                                }
                                frame 2 {
                                n465 = String Subset(string=w1393, offset (0)=3) -> (substring=w1394:string)  [unwired: 1 in]
                                n466 = Hexadecimal String To Number(string=w1394) -> (number=w1392:u32)  [unwired: 2 in, 1 out]
                                n467 = local write "D (Rate) IstWert 2"(w1392) -> ()
                                n468 = local write "D (Rate) Sollwert 2"(w1392) -> ()
                                }
                                frame 3 {
                                n469 = String Subset(string=w1397, offset (0)=3) -> (substring=w1398:string)  [unwired: 1 in]
                                n470 = Hexadecimal String To Number(string=w1398) -> (number=w1396:u32)  [unwired: 2 in, 1 out]
                                n471 = local write "% LOW Istwert 2"(w1396) -> ()
                                n472 = local write "% LOW Sollwert 2"(w1396) -> ()
                                }
                                frame 4 {
                                n473 = String Subset(string=w1401, offset (0)=3) -> (substring=w1402:string)  [unwired: 1 in]
                                n474 = Hexadecimal String To Number(string=w1402) -> (number=w1400:u32)  [unwired: 2 in, 1 out]
                                n475 = local write "% HIGH Istwert 2"(w1400) -> ()
                                n476 = local write "% High Sollwert 2"(w1400) -> ()
                                }
                                frame 5 {
                                n477 = call "I3252_Edit_Setpoint.vi"("Read String"=w1405) -> ("Setpoint is"=w1404:dbl)
                                n478 = local write "SP 2 is (°C)"(w1404) -> ()
                                }
                              }
                            }
                          }
                        }
                      }
                      frame #2 {
                        n479 = property on="RAM 2" class="Bool (strict)"("Blinking"=FALSE) -> ()  [unwired: 2 in, 2 out]
                      }
                    }
                    n480 = Not(x="RAM 2") -> (.not. x?=w1340:bool)
                    n481 = Unbundle(w1338) -> ("VISA resource name out"=w1337:refnum<visa-resource-name>, "error out"=w1336:errorcluster)  [unwired: 2 out]
                  }
                  event "Set Gauge to Zero": Value Change {
                    n482 = event-data() -> ()  [unwired: 1 in, 1 out]
                    n483 = flat-sequence {
                      tunnel: w1414 -> [w1419]
                      tunnel: [w1419] -> w1413
                      tunnel: w1413 -> [w1421]
                      tunnel: [w1425] -> w1412
                      tunnel: [w1424] -> w1411
                      tunnel: [w1421] -> w1410
                      tunnel: w1412 -> [w1431]
                      tunnel: w1411 -> [w1430]
                      tunnel: w1410 -> [w1426]
                      frame #0 {
                        n484 = property on="Set Gauge to Zero" class="Bool"("Blinking"=TRUE) -> ()  [unwired: 2 in, 2 out]
                      }
                      frame #1 {
                        w1422 = 0 items=["sensor 1", "sensor 2", "test"] ("Sensor Nr.:")
                        n485 = call "DUAL GAUGE-Get Pressure,Status.vi"("Sensor Nr.:"=w1422, "Referenz in"=w1421) -> ("Pressure"=w1425:dbl)  [unwired: 6 in, 3 out]
                        n486 = call "DUAL GAUGE-Offset display.vi"("W/R"=FALSE, "Referenz in"=w1421) -> ("Sensor 1 Get"=w1424:dbl)  [unwired: 6 in, 3 out]
                      }
                      frame #2 {
                        n487 = Add(x=w1431, y=w1430) -> (x+y=w1427:dbl)
                        n488 = call "DUAL GAUGE-Offset display.vi"("W/R"=TRUE, "Sensor 1 Set"=w1427, "Referenz in"=w1426) -> ("Sensor 1 Get"=→"Current Offset (mbar)":dbl)  [unwired: 5 in, 3 out]
                      }
                      frame #3 {
                        n489 = property on="Set Gauge to Zero" class="Bool"("Blinking"=TRUE) -> ()  [unwired: 2 in, 2 out]
                      }
                    }
                    n490 = Unbundle(w1418) -> ("VISA resource name out"=w1417:refnum<visa-resource-name>, "error out"=w1416:errorcluster)  [unwired: 2 out]
                    n491 = Unbundle(w1409) -> ("VISA resource name out"=w1408:refnum<visa-resource-name>, "error out"=w1407:errorcluster)  [unwired: 2 out]
                  }
                  event "Write to File": Value Change {
                    n492 = event-data() -> ("NewVal"=w1440:bool)  [unwired: 1 in]
                    n493 = Unbundle(w1443) -> ("VISA resource name out"=w1442:refnum<visa-resource-name>, "error out"=w1441:errorcluster)  [unwired: 2 out]
                    n494 = local read "File Path"() -> (w1436:path)
                    n495 = case shown="False" w1440 {
                      tunnel: w1436 -> [_ w1448]
                      tunnel: "User" -> [_ w1447]
                      tunnel: "Sample" -> [_ w1446]
                      tunnel: [path "" ("File Path") w1445] -> w1437
                      frame False {
                      }
                      frame True {
                        n496 = call "Header.vi"("Sample"=w1446, "User"=w1447, "File Path"=w1448) -> ("File Path"=w1445:path)
                      }
                    }
                    n497 = local write "File Path"(w1437) -> ()
                    n498 = Unbundle(w1435) -> ("VISA resource name out"=w1434:refnum<visa-resource-name>, "error out"=w1433:errorcluster)  [unwired: 2 out]
                  }
                }
              }
              n499 = Bundle(cluster=w418, "VISA resource name out"=w417, "error out"=w416) -> (w415:T7)  [unwired: 2 in]
              n500 = Bundle(cluster=w394, "VISA resource name out"=w396, "error out"=w395) -> (w393:T8)  [unwired: 2 in]
            }
            frame #2 {
            }
            frame #3 {
              (unwired) "Daniel Schuster (geb. 20.03.1988)"
              n501 = node-c288(w1511) -> (w1520:T3)  [unwired: 2 in]
              n502 = node-c288(w1526) -> (w1529:T3)  [unwired: 2 in]
              n503 = node-c288(w1516) -> (w1518:T3)  [unwired: 2 in]
              n504 = node-c288(w1525) -> (w1533:T3)  [unwired: 2 in]
              n505 = timed-sequence {
                timing: w1520 -> [_]
                timing-out: [_] -> w1519
                tunnel: w1495 -> [w1607]
                tunnel: w1494 -> [w1603]
                tunnel: [w1606] -> w1487
                tunnel: w1486 -> [w1605]
                tunnel: w1485 -> [w1604]
                tunnel: [w1602] -> w1484
                tunnel: [w1601] -> w1483
                tunnel: [w1600] -> w1481
                n506 = timed-flat-sequence {
                  tunnel: w1607 -> [w1616]
                  tunnel: [w1615] -> w1606
                  tunnel: w1605 -> [w1614]
                  tunnel: w1604 -> [w1613]
                  tunnel: w1603 -> [w1612]
                  tunnel: [w1610] -> w1602
                  tunnel: [w1609] -> w1601
                  tunnel: [w1608] -> w1600
                  n507 = node-c288() -> ()  [unwired: 1 in, 1 out]
                  n508 = case shown="True" "ON (TPG 2)" {
                    tunnel: w1612 -> [w1621 w1627]
                    tunnel: w1613 -> [w1620 w1626]
                    tunnel: [w1619 w1625] -> w1609
                    tunnel: [w1618 w1624] -> w1608
                    frame False {
                      w1622 = 0.0 ("Pressure")
                      n509 = property on="ON (TPG 2)" class="Bool (strict)"("Blinking"=FALSE) -> ()  [unwired: 2 in, 2 out]
                      n510 = Bundle("Pressure"=w1622, "Pressure"=w1622) -> (w1619:cluster{"Pressure":dbl, "Pressure":dbl})  [unwired: 1 in]
                      n511 = Bundle("TPG 2 COM"=w1621, "error out"=w1620) -> (w1618:T9)  [unwired: 1 in]
                    }
                    frame True {
                      n512 = stacked-sequence {
                        tunnel: w1627 -> [_ w1640]
                        tunnel: [_ w1636] -> w1625
                        tunnel: [_ w1632] -> w1624
                        tunnel: w1626 -> [_ w1629]
                        frame #0 {
                          n513 = property on="ON (TPG 2)" class="Bool (strict)"("Blinking"=TRUE) -> ()  [unwired: 2 in, 2 out]
                        }
                        frame #1 {
                          n514 = call "PresureGetSubVI.vi"("COM in"=w1640, "Fehler (Eingang)"=w1629) -> ("Status Gauge#1"=→"Status Gauge 2#1":i32, "Status Gauge#2"=→"Status Gauge 2#2":i32, "COM out"=w1633:refnum<visa-resource-name>, "Pressure Gauge#1"=w1634:dbl, "Pressure Gauge#2"=w1637:dbl, "Cluster (Ausgang)"=w1630:errorcluster)  [unwired: 12 in]
                          "Pressure Gauge 2#1" <- w1634
                          "Pressure Gauge 2#2" <- w1637
                          n515 = Bundle("COM out"=w1633, "Cluster (Ausgang)"=w1630) -> (w1632:T10)  [unwired: 1 in]
                          n516 = Unbundle(w1630) -> ("status"=w1631:bool, "code"=w1635:i32)  [unwired: 1 out]
                          n517 = Bundle("status"=w1631, "code"=w1635) -> ()  [unwired: 1 in, 1 out]
                          n518 = Bundle("Pressure Gauge#1"=w1634, "Pressure Gauge#2"=w1637) -> (w1636:T11)  [unwired: 1 in]
                        }
                      }
                    }
                  }
                  n519 = case shown="True" "ON (TPG 1)" {
                    tunnel: w1616 -> [w1644 w1650]
                    tunnel: [w1643 w1649] -> w1615
                    tunnel: w1614 -> [w1642 w1648]
                    tunnel: [w1641 w1647] -> w1610
                    frame False {
                      w1645 = 0.0 ("Pressure")
                      n520 = property on="ON (TPG 1)" class="Bool (strict)"("Blinking"=FALSE) -> ()  [unwired: 2 in, 2 out]
                      n521 = Bundle("Pressure"=w1645, "Pressure"=w1645) -> (w1641:cluster{"Pressure":dbl, "Pressure":dbl})  [unwired: 1 in]
                      n522 = Bundle("TPG 1 COM"=w1644, "error out"=w1642) -> (w1643:T12)  [unwired: 1 in]
                    }
                    frame True {
                      n523 = stacked-sequence {
                        tunnel: w1650 -> [_ w1663]
                        tunnel: [_ w1656] -> w1649
                        tunnel: w1648 -> [_ w1653]
                        tunnel: [_ w1652] -> w1647
                        frame #0 {
                          n524 = property on="ON (TPG 1)" class="Bool (strict)"("Blinking"=TRUE) -> ()  [unwired: 2 in, 2 out]
                        }
                        frame #1 {
                          n525 = call "PresureGetSubVI.vi"("COM in"=w1663, "Fehler (Eingang)"=w1653) -> ("Status Gauge#1"=→"Status Gauge 1#1":i32, "Status Gauge#2"=→"Status Gauge 1#2":i32, "COM out"=w1657:refnum<visa-resource-name>, "Pressure Gauge#1"=w1658:dbl, "Pressure Gauge#2"=w1660:dbl, "Cluster (Ausgang)"=w1654:errorcluster)  [unwired: 12 in]
                          "Pressure Gauge 1#1" <- w1658
                          "Pressure Gauge 1#2" <- w1660
                          n526 = Bundle("COM out"=w1657, "Cluster (Ausgang)"=w1654) -> (w1656:T10)  [unwired: 1 in]
                          n527 = Unbundle(w1654) -> ("status"=w1655:bool, "code"=w1659:i32)  [unwired: 1 out]
                          n528 = Bundle("status"=w1655, "code"=w1659) -> ()  [unwired: 1 in, 1 out]
                          n529 = Bundle("Pressure Gauge#1"=w1658, "Pressure Gauge#2"=w1660) -> (w1652:T11)  [unwired: 1 in]
                        }
                      }
                    }
                  }
                  n530 = node-c288() -> ()  [unwired: 1 in, 1 out]
                }
              }
              n531 = timed-sequence {
                timing: w1529 -> [_]
                timing-out: [_] -> w1528
                tunnel: w1527 -> [w1673]
                tunnel: [w1672] -> w1522
                tunnel: [w1671] -> w1521
                tunnel: [w1670] -> w1508
                n532 = timed-flat-sequence {
                  tunnel: w1673 -> [w1677]
                  tunnel: [w1676] -> w1672
                  tunnel: [w1675] -> w1671
                  tunnel: [w1674] -> w1670
                  n533 = node-c288() -> ()  [unwired: 1 in, 1 out]
                  n534 = case shown="True" "ON" {
                    tunnel: w1677 -> [w1681 w1686]
                    tunnel: [w1680 w1685] -> w1676
                    tunnel: [w1679 w1684] -> w1675
                    tunnel: [_ w1683] -> w1674
                    frame False {
                      n535 = Unbundle(w1681) -> ("VISA resource name out"=w1680:refnum<visa-resource-name>, "error out"=w1679:errorcluster)  [unwired: 2 out]
                      n536 = property on="ON" class="Bool (strict)"("Blinking"=FALSE) -> ()  [unwired: 2 in, 2 out]
                    }
                    frame True {
                      n537 = stacked-sequence {
                        tunnel: w1686 -> [_ w1691]
                        tunnel: [_ w1690] -> w1685
                        tunnel: [_ w1689] -> w1684
                        tunnel: [_ w1688] -> w1683
                        frame #0 {
                          n538 = property on="ON" class="Bool (strict)"("Blinking"=TRUE) -> ()  [unwired: 2 in, 2 out]
                        }
                        frame #1 {
                          n539 = Unbundle(w1691) -> ("VISA resource name out"=w1695:refnum<visa-resource-name>, "error out"=w1693:errorcluster, "Delay (ms)"=w1694:u32, "Write/\nRead"=w1692:bool)
                          n540 = call "I3252_Comm_Interface.vi"("VISA resource name in"=w1695, "error in"=w1693, "Delay (ms)"=w1694, "Write"=w1692, "String to Write"="*V01", "Read"=w1692) -> ("VISA resource name out"=w1690:refnum<visa-resource-name>, "error out"=w1689:errorcluster, "Read String"=w1688:string)  [unwired: 2 in]
                        }
                      }
                    }
                  }
                  n541 = node-c288() -> ()  [unwired: 1 in, 1 out]
                }
              }
              n542 = timed-sequence {
                timing: w1518 -> [_]
                timing-out: [_] -> w1517
                tunnel: w1515 -> [w1569]
                tunnel: w1514 -> [w1568]
                tunnel: [w1567] -> w1512
                tunnel: [w1566] -> w1513
                tunnel: [w1565] -> w1509
                n543 = timed-flat-sequence {
                  tunnel: w1569 -> [w1574]
                  tunnel: w1568 -> [w1573]
                  tunnel: [w1572] -> w1567
                  tunnel: [w1571] -> w1566
                  tunnel: [w1570] -> w1565
                  n544 = node-c288() -> ()  [unwired: 1 in, 1 out]
                  n545 = case shown="False" "ON" {
                    tunnel: w1574 -> [w1578 w1584]
                    tunnel: w1573 -> [w1579 w1583]
                    tunnel: [w1578 w1582] -> w1572
                    tunnel: [w1579 w1581] -> w1571
                    tunnel: [0.0 ("Reading") w1580] -> w1570
                    frame False {
                      n546 = property on="ON" class="Bool (strict)"("Blinking"=FALSE) -> ()  [unwired: 2 in, 2 out]
                    }
                    frame True {
                      n547 = stacked-sequence {
                        tunnel: w1584 -> [_ w1591]
                        tunnel: w1583 -> [_ w1590]
                        tunnel: [_ w1589] -> w1582
                        tunnel: [_ w1588] -> w1581
                        tunnel: [_ w1586] -> w1580
                        frame #0 {
                          n548 = property on="ON" class="Bool (strict)"("Blinking"=TRUE) -> ()  [unwired: 2 in, 2 out]
                        }
                        frame #1 {
                          n549 = call "VC840_Read.vi"("error in (no error)"=w1590, "VISA resource name"=w1591) -> ("error out"=w1588:errorcluster, "Unit"=→"Unit 2":string, "Reading"=w1586:dbl, "VISA resource name out"=w1589:refnum<visa-resource-name>, "Status"=→"Status 2":T2, "Mode"=→"Mode 2":enum16{"?", "Diode", "Beep", "DC", "AC"})  [unwired: 4 out]
                          "Reading 2" <- w1586
                        }
                      }
                    }
                  }
                  n550 = node-c288() -> ()  [unwired: 1 in, 1 out]
                }
              }
              n551 = timed-sequence {
                timing: w1533 -> [_]
                timing-out: [_] -> w1532
                tunnel: w1531 -> [w1707]
                tunnel: w1530 -> [w1706]
                tunnel: [w1705] -> w1524
                tunnel: [w1704] -> w1523
                tunnel: [w1703] -> w1510
                n552 = timed-flat-sequence {
                  tunnel: w1707 -> [w1712]
                  tunnel: w1706 -> [w1711]
                  tunnel: [w1710] -> w1705
                  tunnel: [w1709] -> w1704
                  tunnel: [w1708] -> w1703
                  n553 = node-c288() -> ()  [unwired: 1 in, 1 out]
                  n554 = case shown="False" "ON" {
                    tunnel: w1712 -> [w1716 w1722]
                    tunnel: w1711 -> [w1717 w1721]
                    tunnel: [w1716 w1720] -> w1710
                    tunnel: [w1717 w1719] -> w1709
                    tunnel: [0.0 ("Reading") w1718] -> w1708
                    frame False {
                      n555 = property on="ON" class="Bool (strict)"("Blinking"=FALSE) -> ()  [unwired: 2 in, 2 out]
                    }
                    frame True {
                      n556 = stacked-sequence {
                        tunnel: w1722 -> [_ w1729]
                        tunnel: w1721 -> [_ w1728]
                        tunnel: [_ w1727] -> w1720
                        tunnel: [_ w1726] -> w1719
                        tunnel: [_ w1724] -> w1718
                        frame #0 {
                          n557 = property on="ON" class="Bool (strict)"("Blinking"=TRUE) -> ()  [unwired: 2 in, 2 out]
                        }
                        frame #1 {
                          n558 = call "VC840_Read.vi"("error in (no error)"=w1728, "VISA resource name"=w1729) -> ("error out"=w1726:errorcluster, "Unit"=→"Unit 1":string, "Reading"=w1724:dbl, "VISA resource name out"=w1727:refnum<visa-resource-name>, "Status"=→"Status 1":T2, "Mode"=→"Mode 1":enum16{"?", "Diode", "Beep", "DC", "AC"})  [unwired: 4 out]
                          "Reading 1" <- w1724
                        }
                      }
                    }
                  }
                  n559 = node-c288() -> ()  [unwired: 1 in, 1 out]
                }
              }
              n560 = Tick Count (ms)() -> (millisecond timer value=w1496:u32)
              n561 = Subtract(x=w1496, y=w1501) -> (x-y=w1500:u32)
              n562 = Divide(x=w1500, y=u32 1000) -> (x/y=w1498:dbl)
              n563 = node-c288(w1528) -> ()  [unwired: 1 out]
              n564 = node-c288(w1532) -> ()  [unwired: 1 out]
              n565 = node-c288(w1517) -> ()  [unwired: 1 out]
              n566 = node-c288(w1472) -> (w1479:T3)  [unwired: 2 in]
              n567 = To Double Precision Float(number=w1498) -> (double precision float=w1502:dbl)
              "current time (s)" <- w1502
              n568 = timed-sequence {
                timing: w1479 -> [_]
                timing-out: [_] -> w1478
                tunnel: w1477 -> [w1537]
                tunnel: [w1536] -> w1474
                tunnel: [w1535] -> w1473
                tunnel: [w1534] -> w1476
                n569 = timed-flat-sequence {
                  tunnel: w1537 -> [w1542]
                  tunnel: [w1541] -> w1536
                  tunnel: [w1540] -> w1535
                  tunnel: [w1539] -> w1534
                  n570 = node-c288() -> ()  [unwired: 1 in, 1 out]
                  n571 = case shown="True" "ON 2" {
                    tunnel: w1542 -> [w1545 w1549]
                    tunnel: [w1544 w1548] -> w1541
                    tunnel: [w1543 w1547] -> w1540
                    tunnel: [_ w1546] -> w1539
                    frame False {
                      (unwired) FALSE
                      n572 = Unbundle(w1545) -> ("VISA resource name out"=w1544:refnum<visa-resource-name>, "error out"=w1543:errorcluster)  [unwired: 2 out]
                    }
                    frame True {
                      n573 = stacked-sequence {
                        tunnel: w1549 -> [_ w1553]
                        tunnel: [_ w1552] -> w1548
                        tunnel: [_ w1551] -> w1547
                        tunnel: [_ w1550] -> w1546
                        frame #0 {
                          (unwired) TRUE
                        }
                        frame #1 {
                          n574 = Unbundle(w1553) -> ("VISA resource name out"=w1557:refnum<visa-resource-name>, "error out"=w1555:errorcluster, "Delay (ms) 2"=w1556:u32, "Write/\nRead \n\n2"=w1554:bool)
                          n575 = call "I3252_Comm_Interface.vi"("VISA resource name in"=w1557, "error in"=w1555, "Delay (ms)"=w1556, "Write"=w1554, "String to Write"="*V01", "Read"=w1554) -> ("VISA resource name out"=w1552:refnum<visa-resource-name>, "error out"=w1551:errorcluster, "Read String"=w1550:string)  [unwired: 2 in]
                        }
                      }
                    }
                  }
                  n576 = node-c288() -> ()  [unwired: 1 in, 1 out]
                }
              }
              n577 = node-c288(w1519) -> ()  [unwired: 1 out]
              n578 = Unbundle(w1483) -> ("Pressure Gauge#1"=w1482:dbl, "Pressure Gauge#2"=w1480:dbl)
              "Pressure OpenPort2" <- w1480
              "Pressure Pirani 2" <- w1482
              n579 = Unbundle(w1484) -> ("Pressure Gauge#1"=w1493:dbl, "Pressure Gauge#2"=w1488:dbl)
              "Pressure Baratron 2" <- w1493
              "Pressure FullRange 2" <- w1488
              n580 = node-c288(w1478) -> ()  [unwired: 1 out]
            }
            frame #4 {
              n581 = Build Array (concatenate)(w1755, w1759) -> (w1754:dbl[])
              n582 = Build Array (concatenate)(w1758, w1760) -> (w1753:dbl[])
              n583 = Build Array (concatenate)(w1756, w1747) -> (w1751:dbl[])
              n584 = Build Array (concatenate)(w1757, w1748) -> (w1752:dbl[])
              n585 = Greater?(x=w1779, y="Pressure Limit (mbar)") -> (0:w1782:bool)
              n586 = case shown="False" w1782 {
                frame False {
                  w1792 = T6."Enabled" ("Disabled")
                  n587 = property on="Standby" class="Bool (strict)"("DisabledEnum"=w1792) -> ()  [unwired: 2 in, 2 out]
                  n588 = property on="Standby\n2" class="Bool (strict)"("DisabledEnum"=w1792) -> ()  [unwired: 2 in, 2 out]
                }
                frame True {
                  w1794 = T6."Disabled" ("Disabled")
                  w1793 = TRUE ("Standby")
                  n589 = property on="Standby" class="Bool (strict)"("Val(Sgnl)"=w1793, "DisabledEnum"=w1794) -> ()  [unwired: 2 in, 2 out]
                  n590 = property on="Standby\n2" class="Bool (strict)"("Val(Sgnl)"=w1793, "DisabledEnum"=w1794) -> ()  [unwired: 2 in, 2 out]
                }
              }
              n591 = call "Resistivity_Calculation.vi"("Reading 1 (V)"=w1772, "Constant"="4PP constant", "Thickness (nm)"="Thickness (nm)", "Reading 2 (A)"=w1780) -> ("Resivtivity (Ohm*cm)"=w1764:dbl, "Current"=w1765:dbl, "Voltage"=w1766:dbl)
              "Resistivity (Ohm*cm)" <- w1764
              "Voltage (V)" <- w1766
              "Current (A)" <- w1765
              n592 = call "I3252_Edit_Temperature.vi"("Temp. String"=w1781) -> ("Temp. (°C)"=w1775:dbl)
              "(°C)" <- w1775
              n593 = call "I3252_Edit_Temperature.vi"("Temp. String"=w1743) -> ("Temp. (°C)"=w1742:dbl)
              "(°C) 2" <- w1742
              n594 = Build Array (concatenate)(w1777, w1778) -> (w1774:dbl[])
              n595 = Build Array (concatenate)(w1776, w1775) -> (w1762:dbl[])
              n596 = Build Array (concatenate)(w1740, w1742) -> (w1741:dbl[])
              n597 = Build Array (concatenate)(w1773, w1766) -> (w1771:dbl[])
              n598 = Build Array (concatenate)(w1770, w1765) -> (w1768:dbl[])
              n599 = Build Array (concatenate)(w1769, w1764) -> (w1767:dbl[])
              n600 = Build Array(w1766, w1765, w1764) -> (w1763:dbl[])
            }
            frame #5 {
              n601 = Bundle(w1797, w1814) -> (→"CMR275 Baratron":cluster{dbl[], dbl[]})  [unwired: 1 in]
              n602 = Bundle(w1797, w1813) -> (→"PKR251 FullRange":cluster{dbl[], dbl[]})  [unwired: 1 in]
              n603 = Bundle(w1797, w1812) -> (→"Pirani (VVP1 Scroll)":cluster{dbl[], dbl[]})  [unwired: 1 in]
              n604 = Bundle(w1797, w1811) -> (→"Pressure OpenPort":cluster{dbl[], dbl[]})  [unwired: 1 in]
              n605 = Bundle(w1797, w1820) -> (→"Thermocouple (Sample holder 1)":cluster{dbl[], dbl[]})  [unwired: 1 in]
              n606 = Bundle(w1797, w1822) -> (→"Voltage":cluster{dbl[], dbl[]})  [unwired: 1 in]
              n607 = Bundle(w1797, w1823) -> (→"Current":cluster{dbl[], dbl[]})  [unwired: 1 in]
              n608 = Bundle(w1797, w1824) -> (→"Resistivity":cluster{dbl[], dbl[]})  [unwired: 1 in]
              n609 = Bundle(w1797, w1798) -> (→"Thermocouple (Sample holder 1) 2":cluster{dbl[], dbl[]})  [unwired: 1 in]
              n610 = Build Array (concatenate)(w1819, w1829, w1828, w1818, w1806, w1802, w1800) -> (w1836:dbl[])
              "appended array" <- w1836
            }
            frame #6 {
              n611 = Unbundle(w1845) -> ("COM out"=w1844:refnum<visa-resource-name>, "Cluster (Ausgang)"=w1843:errorcluster)
              n612 = Unbundle(w1842) -> ("COM out"=w1841:refnum<visa-resource-name>, "Cluster (Ausgang)"=w1840:errorcluster)
              n613 = case shown="True" "Write to File" {
                tunnel: [_ w1873] -> w1859
                tunnel: "File Path" -> [_ w1871]
                tunnel: w1852 -> [_ w1869]
                frame False {
                  n614 = property on="Write to File" class="Bool (strict)"("Blinking"=FALSE) -> ()  [unwired: 2 in, 2 out]
                }
                frame True {
                  n615 = flat-sequence {
                    tunnel: [w1875] -> w1872
                    tunnel: w1871 -> [w1875]
                    tunnel: [w1874] -> w1870
                    tunnel: w1869 -> [w1874]
                    tunnel: [w1880] -> w1873
                    tunnel: w1872 -> [w1879]
                    tunnel: w1870 -> [w1878]
                    frame #0 {
                      n616 = property on="Write to File" class="Bool (strict)"("Blinking"=TRUE) -> ()  [unwired: 2 in, 2 out]
                    }
                    frame #1 {
                      n617 = call-poly <vilib>:"Write To Spreadsheet File.vi"("format (%.3f)"="%g", "append to file? (new file:F)"=TRUE ("transpose? (no:F)"), "1D data"=w1878, "file path (dialog if empty)"=w1879) -> ("new file path (Not A Path if cancelled)"=w1880:path)  [unwired: 4 in]
                    }
                  }
                }
              }
              n618 = Merge Errors(w1864, w1863, w1861, w1843, w1840) -> (w1862:errorcluster)
              n619 = call <vilib>:"Simple Error Handler.vi"("error in (no error)"=w1862) -> ("error?"=w1846:bool)  [unwired: 4 in, 4 out]
              n620 = local write "File Path"(w1859) -> ()
            }
            frame #7 {
              w1899 = u32 1000 ("y")
              n621 = Tick Count (ms)() -> (millisecond timer value=w1901:u32)
              n622 = Subtract(x=w1901, y=w1900) -> (x-y=w1902:u32)
              n623 = VISA Flush I/O Buffer(VISA resource name=w1893, error in (no error)=w1892) -> (VISA resource name out=w1890:refnum<visa-resource-name>, error out=w1891:errorcluster)  [unwired: 1 in]
              n624 = VISA Flush I/O Buffer(VISA resource name=w1886, error in (no error)=w1885) -> (VISA resource name out=w1889:refnum<visa-resource-name>, error out=w1888:errorcluster)  [unwired: 1 in]
              n625 = Divide(x=w1902, y=w1899) -> (x/y=→"loop time (s)":dbl)
              n626 = Subtract(x="Intervall (s)", y=u32 1) -> (x-y=w1903:u32)
              n627 = Multiply(x=w1903, y=w1899) -> (x*y=w1906:u32)
              n628 = Wait (ms)(milliseconds to wait=w1906) -> ()  [unwired: 1 out]
              n629 = Bundle("COM out"=w1890, "error out"=w1891, "COM out"=w1889, "error out"=w1888) -> (w1887:T13)  [unwired: 1 in]
            }
            frame #8 {
              n630 = Tick Count (ms)() -> (millisecond timer value=w1929:u32)
              n631 = Subtract(x=w1929, y=w1927) -> (x-y=w1928:u32)
              n632 = Divide(x=w1928, y=w1926) -> (x/y=→"data logger intervall (s)":dbl)
            }
          }
          n633 = Exclusive Or(1:"stop", 2:w175) -> (0:w176:bool)
        }
      }
      frame #4 {
        n634 = call "VC840_Close.vi"("error in (no error)"=w1951, "VISA resource name"=w1952) -> ("error out"=w1960:errorcluster)  [unwired: 9 in]
        n635 = call "VC840_Close.vi"("error in (no error)"=w1953, "VISA resource name"=w1954) -> ("error out"=w1958:errorcluster)  [unwired: 9 in]
        n636 = VISA Close(VISA resource name=w1956, error in (no error)=w1955) -> (error out=w1957:errorcluster)
        n637 = VISA Close(VISA resource name=w1944, error in (no error)=w1943) -> (error out=w1942:errorcluster)
        n638 = Unbundle(w1949) -> ("COM out"=w1948:refnum<visa-resource-name>, "error out"=w1947:errorcluster, "COM out"=w1945:refnum<visa-resource-name>, "error out"=w1946:errorcluster)
        n639 = VISA Close(VISA resource name=w1948, error in (no error)=w1947) -> ()  [unwired: 1 out]
        n640 = VISA Close(VISA resource name=w1945, error in (no error)=w1946) -> ()  [unwired: 1 out]
        n641 = Merge Errors(w1957, w1958, w1960, w1942) -> (w1959:errorcluster)
        n642 = call <vilib>:"Simple Error Handler.vi"("error in (no error)"=w1959) -> ("error?"=w1950:bool)  [unwired: 1 in, 7 out]
        n643 = Stop(stop? (T)=w1950) -> ()
      }
    }
  }
